vi "运维调试_质控单元.vi"() -> ()   [LabVIEW 2016, in "质控单元.lvlib"]
uses:
  <vilib>/Utility/miscctls.llb/LVPointTypeDef.ctl
  <vilib>/Utility/config.llb/Read Key (I32).vi
  <vilib>/Utility/config.llb/Read Key (Boolean).vi
  <vilib>/Utility/config.llb/Read Key (U32).vi
  <vilib>/Utility/config.llb/Write Key (I32).vi
  <vilib>/Utility/config.llb/Write Key (Boolean).vi
  <vilib>/Utility/config.llb/NI_LVConfig.lvlib
panel:
  in  "定时启动":bool
  out "CODCr母液浓度":dbl caption="加标母液浓度" format="%.2f"
  out "CODCr加标水杯定容体积":dbl caption="加标水杯定容体积" format="%.2f"
  out "CODCr检出限":dbl caption="检出限" format="%.2f"
  out "CODCr量程":dbl caption="量程" format="%.2f"
  out "COD母液浓度":dbl caption="加标母液浓度" format="%.2f"
  out "COD加标水杯定容体积":dbl caption="加标水杯定容体积" format="%.2f"
  out "COD检出限":dbl caption="检出限" format="%.2f"
  out "COD量程":dbl caption="量程" format="%.2f"
  out "总氮母液浓度":dbl caption="加标母液浓度" format="%.3f"
  out "总氮加标水杯定容体积":dbl caption="加标水杯定容体积" format="%.2f"
  out "总氮检出限":dbl caption="检出限" format="%.3f"
  out "总氮量程":dbl caption="量程" format="%.2f"
  out "总磷母液浓度":dbl caption="加标母液浓度" format="%.3f"
  out "总磷加标水杯定容体积":dbl caption="加标水杯定容体积" format="%.2f"
  out "总磷检出限":dbl caption="检出限" format="%.3f"
  out "总磷量程":dbl caption="量程" format="%.2f"
  out "氨氮母液浓度":dbl caption="加标母液浓度" format="%.3f"
  out "氨氮加标水杯定容体积":dbl caption="加标水杯定容体积" format="%.2f"
  out "氨氮检出限":dbl caption="检出限" format="%.3f"
  out "氨氮量程":dbl caption="量程" format="%.2f"
  in  "释放串口":bool
  in  "打开串口":bool
  out "CODCr质控流程中":bool
  out "CODMn质控流程中":bool
  out "总磷质控流程中":bool
  out "总氮质控流程中":bool
  out "氨氮质控流程中":bool
  out "CODCr通讯":bool
  out "CODMn通讯":bool
  out "总磷总氮通讯":bool
  out "氨氮通讯":bool
  out "CODCr传感器状态显示":bool
  out "CODCr超时报警":bool
  out "CODMn超时报警":bool
  out "总磷总氮超时报警":bool
  out "氨氮进样超时报警":bool
  out "CODMn传感器状态显示":bool
  out "总磷总氮传感器状态显示":bool
  out "氨氮传感器状态显示":bool
  out "CODCr流程中断报警":bool
  out "总磷总氮流程中断报警":bool
  out "CODMn流程中断报警":bool
  out "氨氮流程中断报警":bool
  in  "手动调试":bool
  in  "报警清除":bool
  in  "查看":bool
  in  "停止测量":bool
  in  "加标回收":bool
  in  "平行样测试":bool
  in  "CODCr量程选择":enum32{"H", "L", "AUTO"}(ring)
  in  "CODCr选择":bool
  out "CODCr加标回收率":dbl caption="加标回收率" format="%.2f"
  out "CODCr加标体积":dbl caption="加标体积" format="%.3f"
  out "CODCr加标后水样浓度":dbl caption="加标后水样浓度" format="%.2f"
  out "CODCr加标前水样浓度":dbl caption="加标前水样浓度" format="%.2f"
  out "CODCr状态":u16(ring) caption="状态" items=["待机", "润洗", "进样", "等待取液", "排液"]
  out "质控流程中":bool
  in  "CODMn量程选择":enum32{"H", "L", "AUTO"}(ring)
  in  "总磷量程选择":enum32{"H", "L", "AUTO"}(ring)=enum."AUTO"
  in  "总氮量程选择":enum32{"H", "L", "AUTO"}(ring)=enum."AUTO"
  in  "氨氮量程选择":enum32{"H", "L", "AUTO"}(ring)=enum."AUTO"
  in  "CODMn选择":bool
  in  "总磷总氮模块选择":bool
  in  "氨氮模块":bool
  in  "背隙补偿步数 3":i32 min=0 max=2000
  in  "背隙补偿步数 2":i32 min=0 max=2000
  in  "背隙补偿步数":i32 min=0 max=2000
  out "总氮加标回收率":dbl caption="加标回收率" format="%.2f"
  out "总氮加标体积":dbl caption="加标体积" format="%.3f"
  out "总氮加标后水样浓度":dbl caption="加标后水样浓度" format="%.3f"
  out "总氮加标前水样浓度":dbl caption="加标前水样浓度" format="%.3f"
  out "总氮状态":u16(ring) caption="状态" items=["待机", "润洗", "进样", "等待取液", "排液"]
  in  "返回":bool
  out "COD加标回收率":dbl caption="加标回收率" format="%.2f"
  out "COD加标体积":dbl caption="加标体积" format="%.3f"
  out "COD加标后水样浓度":dbl caption="加标后水样浓度" format="%.2f"
  out "COD加标前水样浓度":dbl caption="加标前水样浓度" format="%.2f"
  out "CODMn状态":u16(ring) caption="状态" items=["待机", "润洗", "进样", "等待取液", "排液"]
  out "总磷加标回收率":dbl caption="加标回收率" format="%.2f"
  out "总磷加标体积":dbl caption="加标体积" format="%.3f"
  out "总磷加标后水样浓度":dbl caption="加标后水样浓度" format="%.3f"
  out "总磷加标前水样浓度":dbl caption="加标前水样浓度" format="%.3f"
  out "总磷状态":u16(ring) caption="状态" items=["待机", "润洗", "进样", "等待取液", "排液"]
  out "氨氮加标回收率":dbl caption="加标回收率" format="%.2f"
  out "氨氮加标体积":dbl caption="加标体积" format="%.3f"
  out "氨氮加标后水样浓度":dbl caption="加标后水样浓度" format="%.3f"
  out "氨氮加标前水样浓度":dbl caption="加标前水样浓度" format="%.3f"
  out "氨氮状态":u16(ring) caption="状态" items=["待机", "润洗", "进样", "等待取液", "排液"]
  # "氨氮"
  # "总磷"
  # "总氮"
  # "CODMn"
  # "CODCr"
  # "参数配置区"
  # "2000步等于1mL\n100步等于0.05mL\n20步等于0.01mL\n2步等于0.001mL\n（初始默认100步）"
  # "CODCr质控参数"
  # "mg/L"
  # "mL"
  # "mg/L"
  # "mg/L"
  # "CODMn质控参数"
  # "mg/L"
  # "mL"
  # "mg/L"
  # "mg/L"
  # "总氮质控参数"
  # "mg/L"
  # "mL"
  # "mg/L"
  # "mg/L"
  # "总磷质控参数"
  # "mg/L"
  # "mL"
  # "mg/L"
  # "mg/L"
  # "氨氮质控参数"
  # "mg/L"
  # "mL"
  # "mg/L"
  # "mg/L"
  # "%"
  # "mL"
  # "mg/L"
  # "mg/L"
  # "%"
  # "mL"
  # "mg/L"
  # "mg/L"
  # "%"
  # "mL"
  # "mg/L"
  # "mg/L"
  # "%"
  # "mL"
  # "mg/L"
  # "mg/L"
  # "%"
  # "mL"
  # "mg/L"
  # "mg/L"
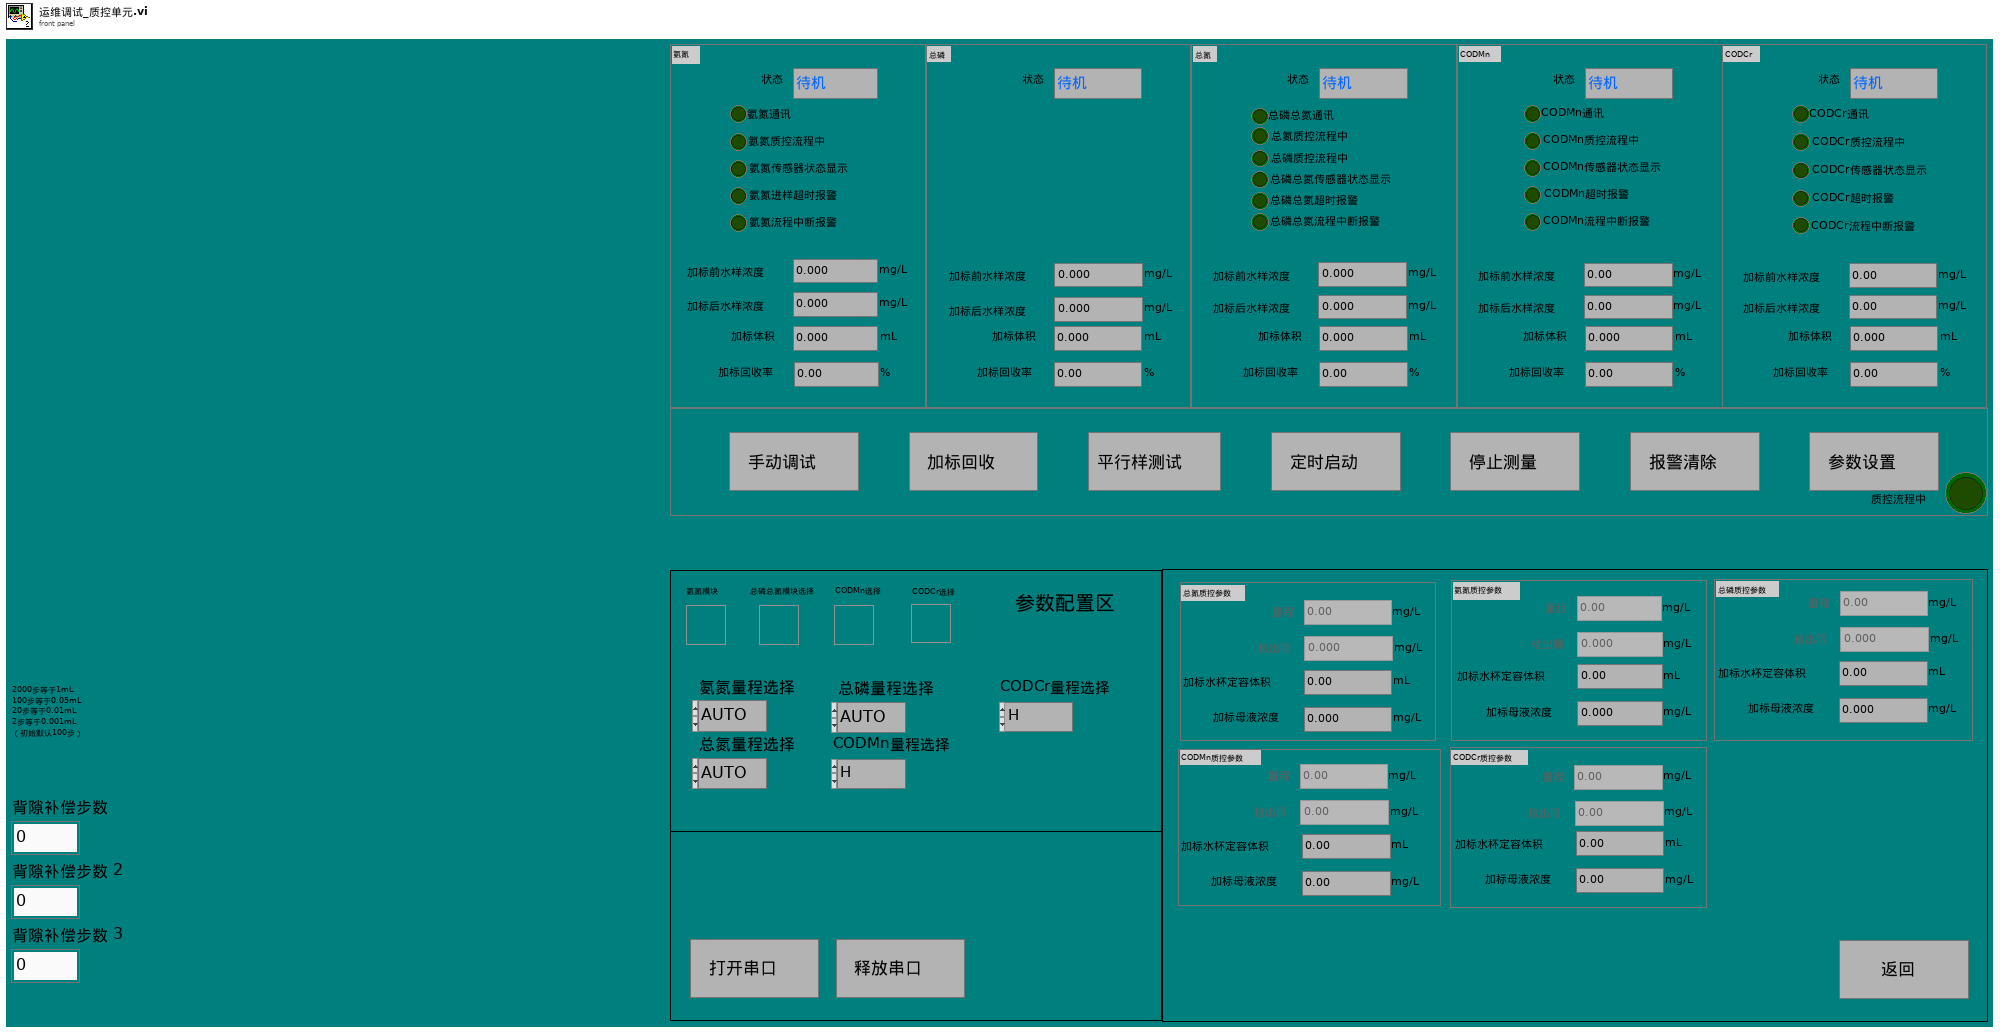
[diagram p1: front panel]
types:
  T1 = typedef "LVPointTypeDef.ctl" = cluster{"Horizontal":i16, "Vertical":i16}
  T2 = typedef "NI_LVConfig.lvlib/Config Data RefNum.ctl" = refnum<k1>
  T3 = cluster{"量程":dbl, "检出限":dbl, "加标前水样浓度":dbl, "加标后水样浓度":dbl, "加标水杯定容体积":dbl, "加标母液浓度":dbl, "加标体积":dbl, "加标回收率":dbl}
  T4 = enum8{"Enabled", "Disabled", "Disabled and Grayed Out"}
  T5 = cluster{"是否启用仪器":bool, "CODMn":cluster{"启动测量模式":cluster{"测量模式":enum16{"水样测量", "标样核查", "加标回收", "平行样", "校零", "校标"}}, "确定按钮":bool}, "启动模块":cluster{"氨氮":bool, "总磷":bool, "总氮":bool, "CODMn":bool, "CODCr":bool}, "常规启动":bool, "直接启动":bool}
  T6 = cluster{"参数启用":cluster{"CODMn":bool, "总磷":bool, "总氮":bool, "氨氮":bool, "CODcr":bool}, "采配水是否启动":bool}
  T7 = cluster{"命令":string, cluster{"starting address":u16, "holding register value":u16}}
  T8 = cluster{"周期设置类型":enum16{"定点启动", "间隔启动"}, "定时功能启用":bool, "定时间隔":dbl, "间隔启动次数 ":dbl, "已经启动次数 ":dbl, "24H周期设置":bool[], "模块选择":cluster{"氨氮":bool, "总磷":bool, "总氮":bool, "CODMn":bool, "CODCr":bool}, "采配水启用":bool}
  T9 = cluster{"周期设置类型":enum16{"定点启动", "间隔启动"}, "定时功能启用":bool, "定时间隔":dbl, "间隔启动次数":dbl, "已经启动次数":dbl, "24H周期设置":bool[], "模块选择":cluster{"氨氮":bool, "总磷":bool, "总氮":bool, "CODMn":bool, "CODCr":bool}, "采配水启用":bool}
  T10 = cluster{"氨氮":bool, "总磷":bool, "总氮":bool, "CODMn":bool, "CODCr":bool}
  T11 = enum32{"Bad", "Idle", "Run top level", "Running"}
  T12 = cluster{"CODMn":bool, "总磷":bool, "总氮":bool, "氨氮":bool, "CODCr":bool}
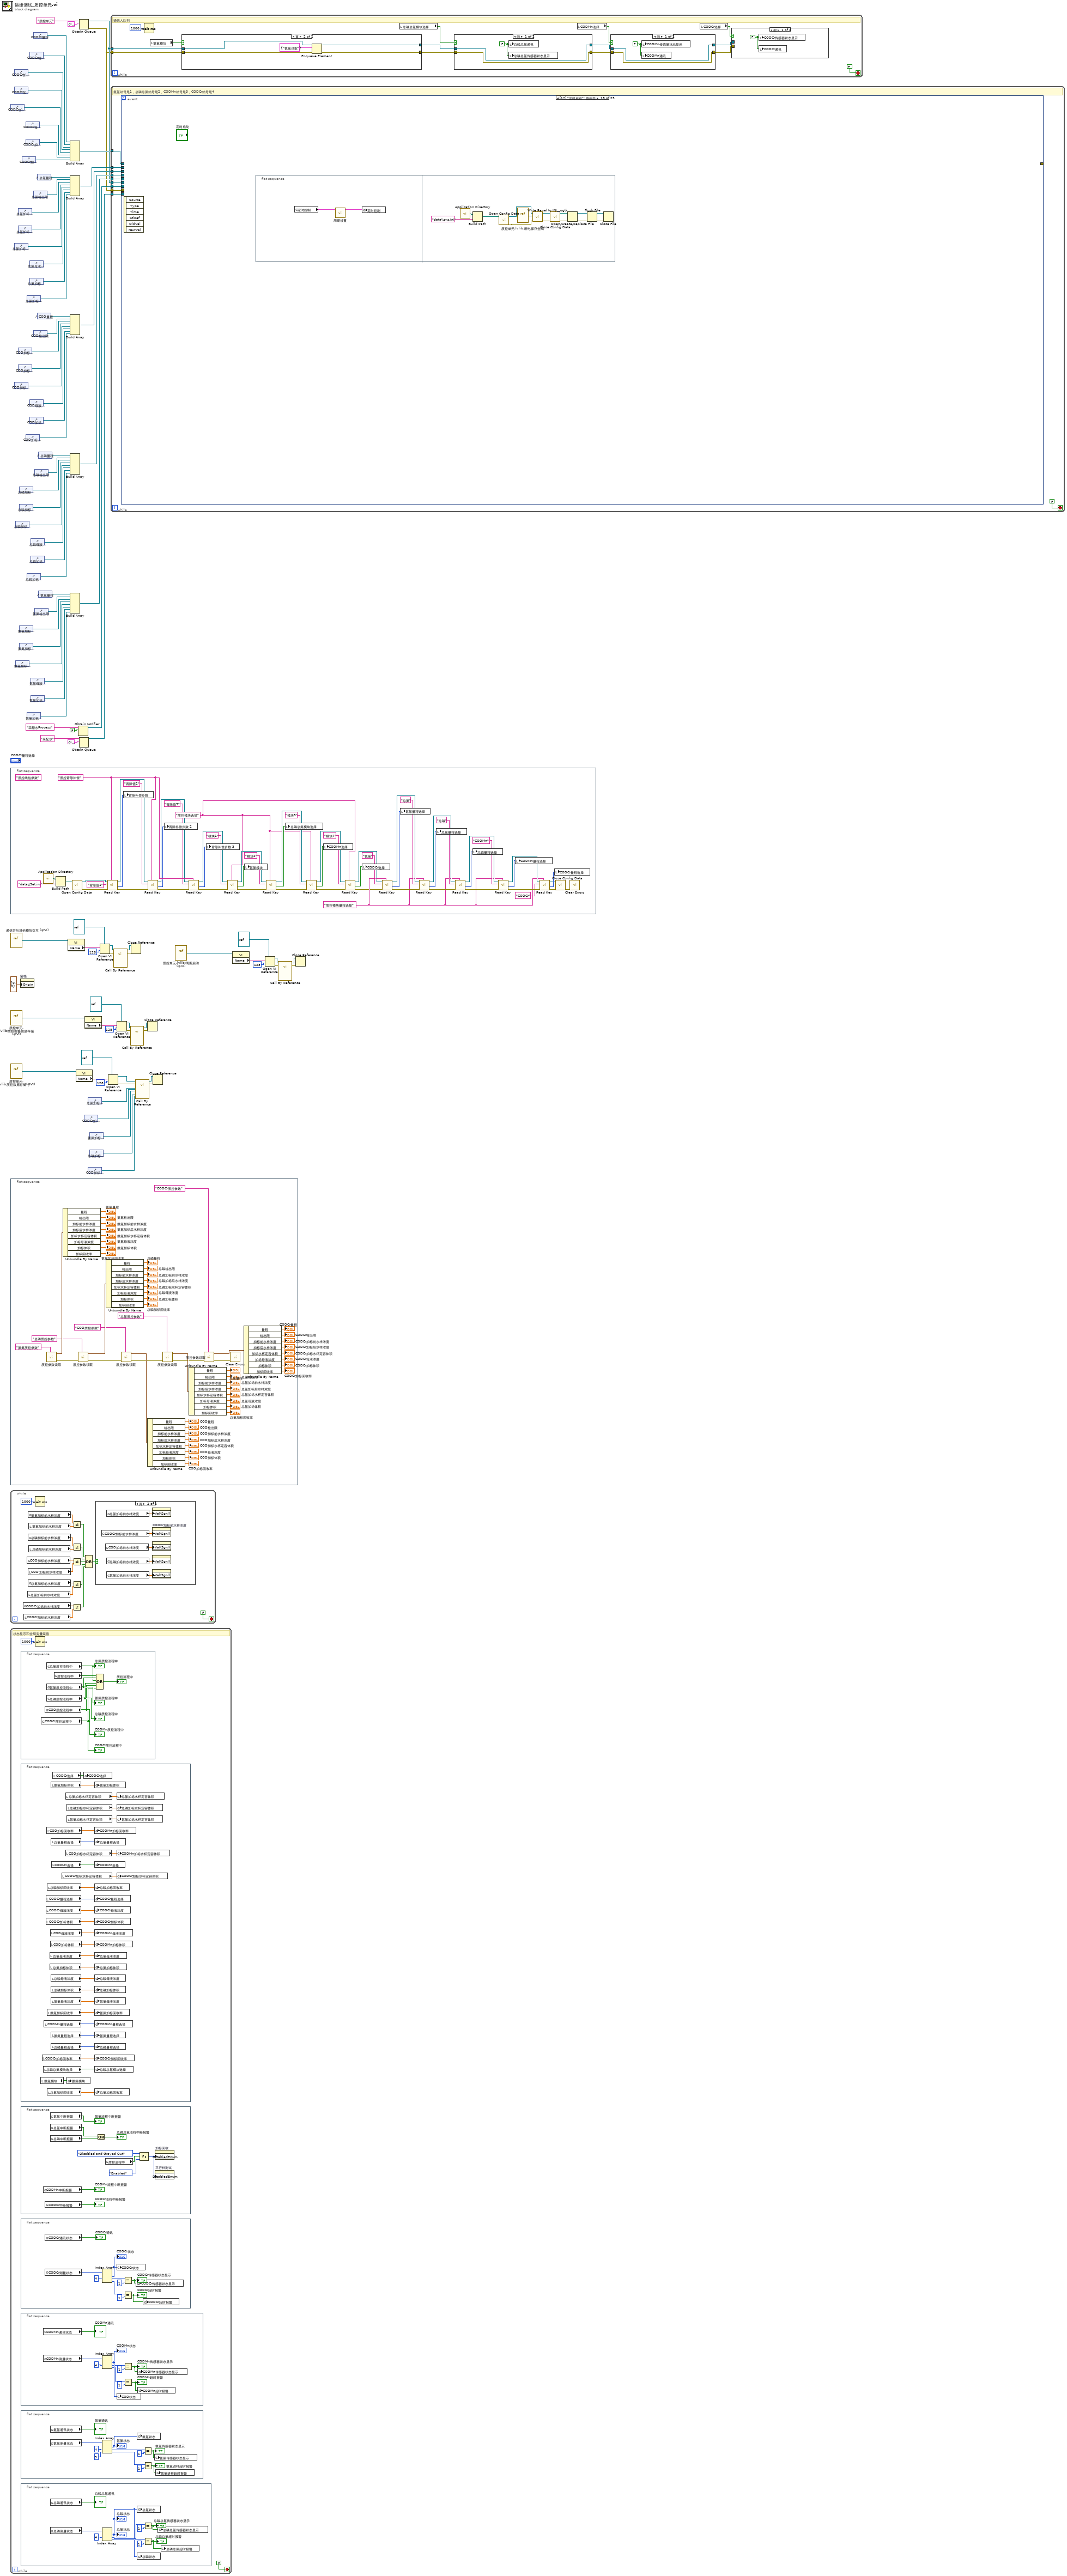
[diagram p0: block diagram]
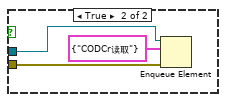
[diagram p2: hidden frame]
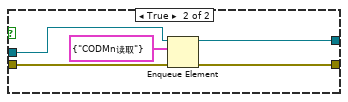
[diagram p3: hidden frame]
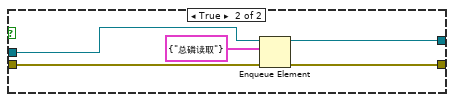
[diagram p4: hidden frame]
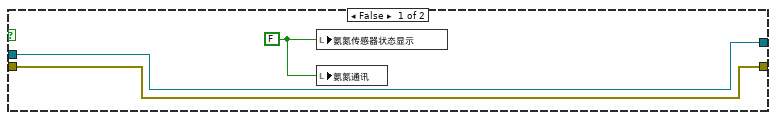
[diagram p5: hidden frame]
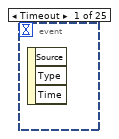
[diagram p7: hidden frame]
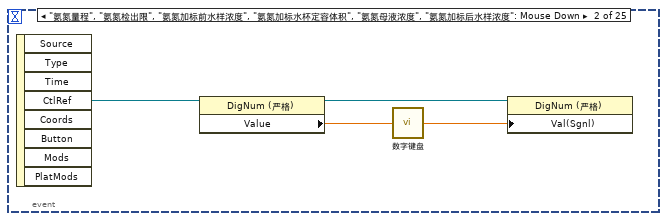
[diagram p8: hidden frame]
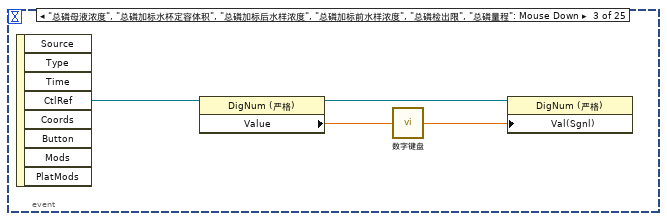
[diagram p9: hidden frame]
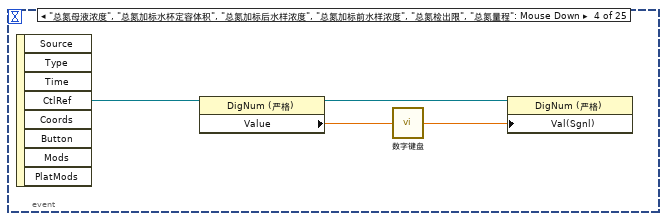
[diagram p10: hidden frame]
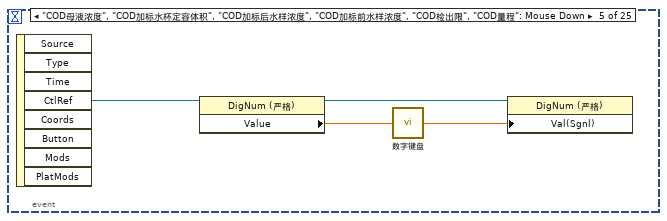
[diagram p11: hidden frame]
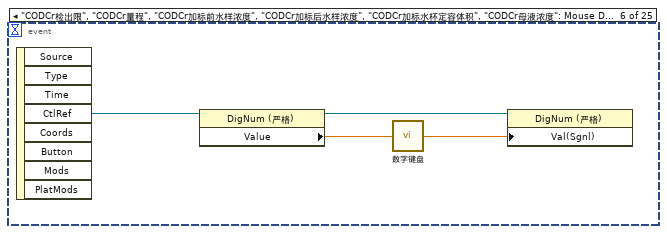
[diagram p12: hidden frame]
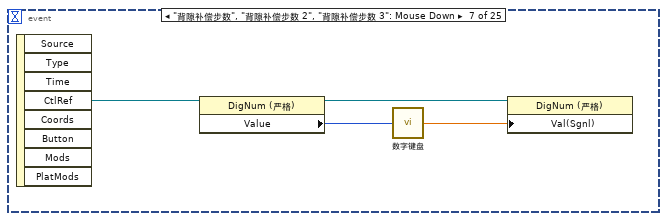
[diagram p13: hidden frame]
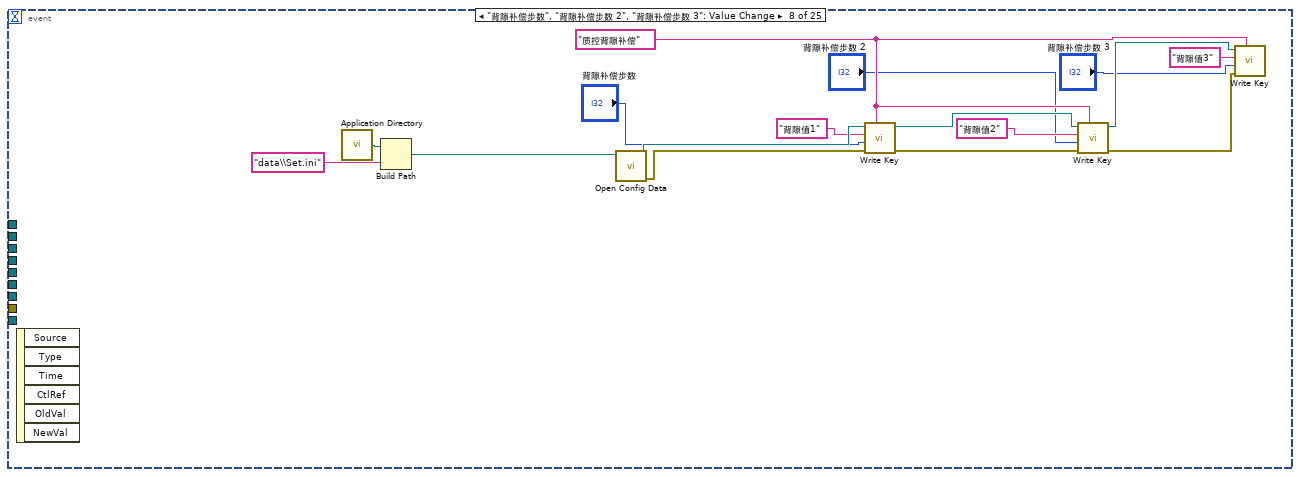
[diagram p14: hidden frame]
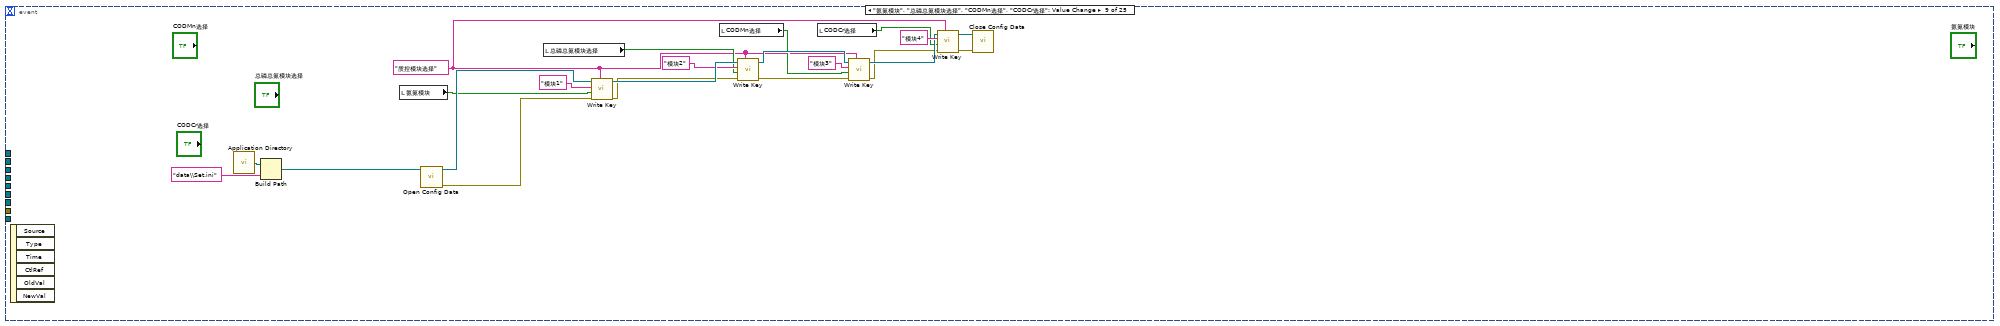
[diagram p15: hidden frame]
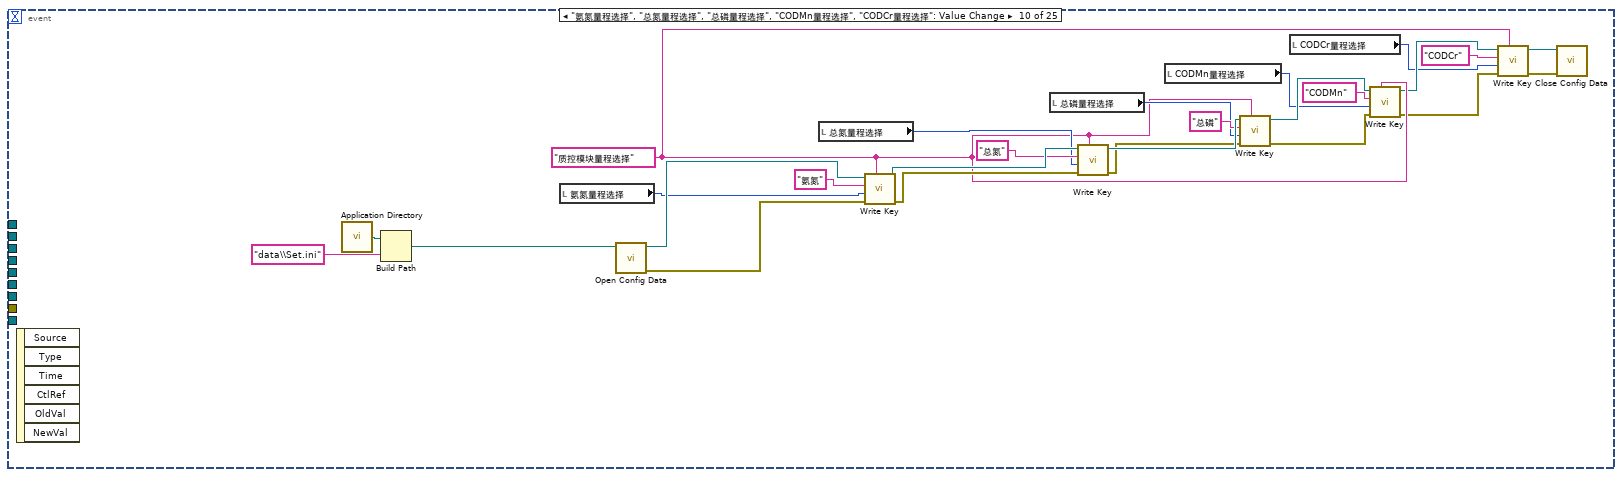
[diagram p16: hidden frame]
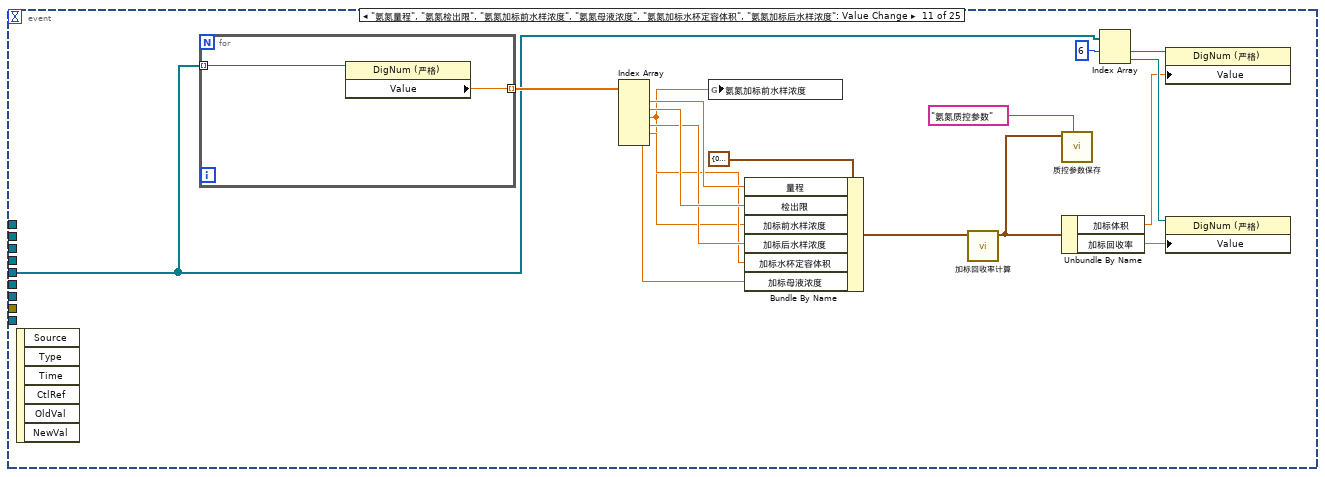
[diagram p17: hidden frame]
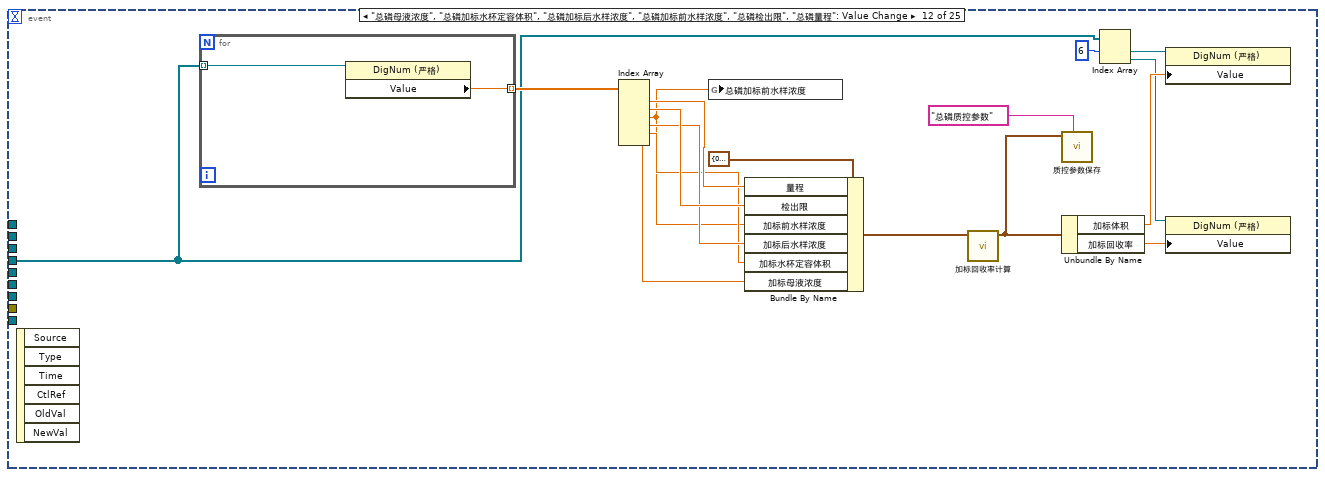
[diagram p18: hidden frame]
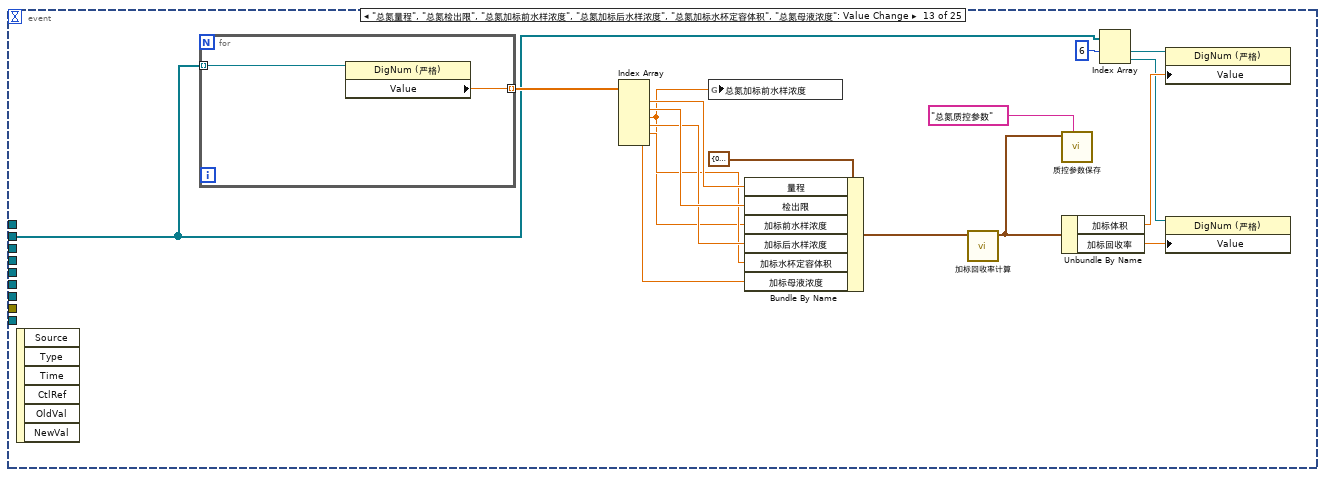
[diagram p19: hidden frame]
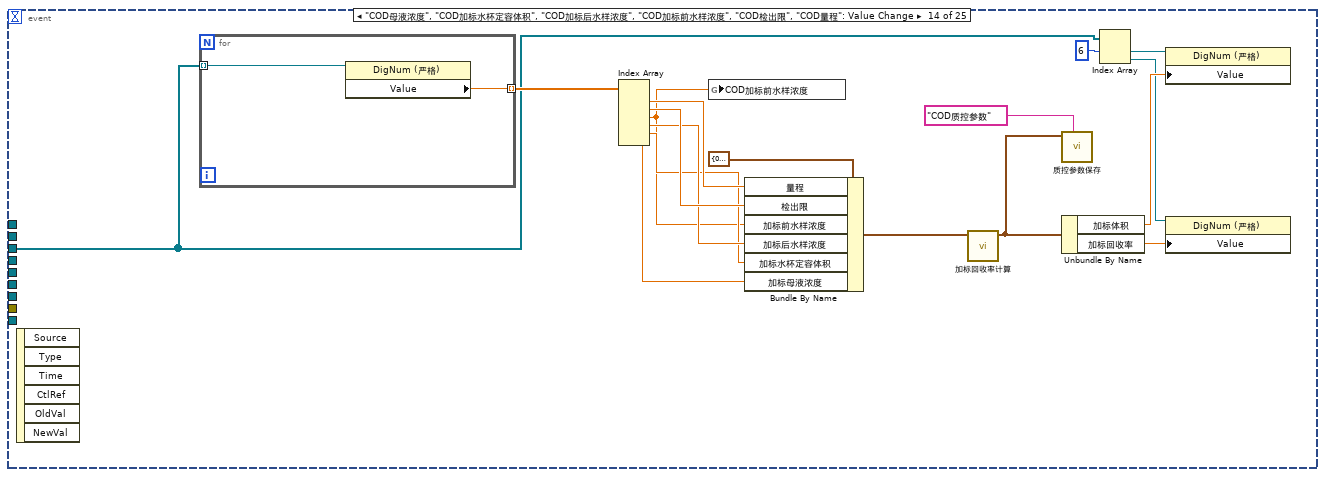
[diagram p20: hidden frame]
diagram:
  n1 = control-ref of="CODCr加标水杯定容体积"() -> (w46:refnum<vi>)
  n2 = flat-sequence {
    frame #0 {
      w108 = "质控模块量程选择" ("section")
      w100 = "质控模块选择" ("section")
      (unwired) "质控线性参数" ("section")
      w144 = "质控背隙补偿" ("section")
      n3 = call <vilib>:"Application Directory.vi"() -> ("Application Directory"=w150:path)
      n4 = Build Path(base path=w150, name or relative path="data\\Set.ini" ("名称或相对路径")) -> (appended path=w148:path)
      n5 = call <vilib>:"Open Config Data.vi"("configuration file path"=w148) -> ("error out"=w146:errorcluster, "refnum"=w147:T2)  [unwired: 8 in, 1 out]
      n6 = call-poly <vilib>:"Read Key.vi"("section"=w144, "error in (no error)"=w146, "key"="背隙值1", "refnum"=w147) -> ("error out"=w141:errorcluster, "value"=w136:i32, "refnum out"=w143:T2)  [unwired: 4 in, 1 out]
      n7 = local write "背隙补偿步数"(w136) -> ()
      n8 = call-poly <vilib>:"Read Key.vi"("section"=w144, "error in (no error)"=w141, "key"="背隙值2", "refnum"=w143) -> ("error out"=w139:errorcluster, "value"=w137:i32, "refnum out"=w140:T2)  [unwired: 4 in, 1 out]
      n9 = local write "背隙补偿步数 2"(w137) -> ()
      n10 = call-poly <vilib>:"Read Key.vi"("section"=w144, "error in (no error)"=w139, "key"="背隙值3", "refnum"=w140) -> ("error out"=w95:errorcluster, "value"=w135:i32, "refnum out"=w96:T2)  [unwired: 4 in, 1 out]
      n11 = local write "背隙补偿步数 3"(w135) -> ()
      n12 = call-poly <vilib>:"Read Key.vi"("section"=w100, "error in (no error)"=w95, "key"="模块1" ("section"), "refnum"=w96) -> ("error out"=w133:errorcluster, "value"=w125:bool, "refnum out"=w134:T2)  [unwired: 4 in, 1 out]
      n13 = local write "氨氮模块"(w125) -> ()
      n14 = call-poly <vilib>:"Read Key.vi"("section"=w100, "error in (no error)"=w133, "key"="模块2" ("section"), "refnum"=w134) -> ("error out"=w131:errorcluster, "value"=w126:bool, "refnum out"=w132:T2)  [unwired: 4 in, 1 out]
      n15 = local write "总磷总氮模块选择"(w126) -> ()
      n16 = call-poly <vilib>:"Read Key.vi"("section"=w100, "error in (no error)"=w131, "key"="模块3" ("section"), "refnum"=w132) -> ("error out"=w102:errorcluster, "value"=w127:bool, "refnum out"=w103:T2)  [unwired: 4 in, 1 out]
      n17 = local write "CODMn选择"(w127) -> ()
      n18 = call-poly <vilib>:"Read Key.vi"("section"=w100, "error in (no error)"=w102, "key"="模块4", "refnum"=w103) -> ("error out"=w98:errorcluster, "value"=w97:bool, "refnum out"=w99:T2)  [unwired: 4 in, 1 out]
      n19 = local write "CODCr选择"(w97) -> ()
      n20 = call-poly <vilib>:"Read Key.vi"("section"=w108, "error in (no error)"=w98, "key"="氨氮" ("section"), "refnum"=w99) -> ("error out"=w123:errorcluster, "value"=w114:u32, "refnum out"=w124:T2)  [unwired: 4 in, 1 out]
      n21 = local write "氨氮量程选择"(w114) -> ()
      n22 = call-poly <vilib>:"Read Key.vi"("section"=w108, "error in (no error)"=w123, "key"="总氮" ("section"), "refnum"=w124) -> ("error out"=w121:errorcluster, "value"=w113:u32, "refnum out"=w122:T2)  [unwired: 4 in, 1 out]
      n23 = local write "总氮量程选择"(w113) -> ()
      n24 = call-poly <vilib>:"Read Key.vi"("section"=w108, "error in (no error)"=w121, "key"="总磷" ("section"), "refnum"=w122) -> ("error out"=w119:errorcluster, "value"=w112:u32, "refnum out"=w120:T2)  [unwired: 4 in, 1 out]
      n25 = local write "总磷量程选择"(w112) -> ()
      n26 = call-poly <vilib>:"Read Key.vi"("section"=w108, "error in (no error)"=w119, "key"="CODMn" ("section"), "refnum"=w120) -> ("error out"=w109:errorcluster, "value"=w111:u32, "refnum out"=w110:T2)  [unwired: 4 in, 1 out]
      n27 = local write "CODMn量程选择"(w111) -> ()
      n28 = call-poly <vilib>:"Read Key.vi"("section"=w108, "error in (no error)"=w109, "key"="CODCr" ("section"), "refnum"=w110) -> ("error out"=w105:errorcluster, "value"=w106:u32, "refnum out"=w104:T2)  [unwired: 4 in, 1 out]
      n29 = local write "CODCr量程选择"(w106) -> ()
      n30 = call <vilib>:"Close Config Data.vi"("error in (no error)"=w105, "refnum"=w104) -> ("error out"=w94:errorcluster)  [unwired: 8 in, 1 out]
      n31 = call <vilib>:"Clear Errors.vi"("error in (no error)"=w94) -> ()  [unwired: 5 in, 2 out]
    }
  }
  n32 = vi-ref "通信并与其他模块交互 (子VI).vi"() -> (w34:refnum<vi>)
  n33 = vi-ref "质控单元.lvlib:质控报警信息存储 (子VI).vi"() -> (w29:refnum<vi>)
  n34 = vi-ref "质控单元.lvlib:质控数据存储(子VI).vi"() -> (w14:refnum<vi>)
  n35 = flat-sequence {
    frame #0 {
      n36 = call "质控参数读取.vi"("section"="氨氮质控参数") -> ("error out"=w185:errorcluster, "参数"=w204:T3)  [unwired: 9 in]
      n37 = Unbundle By Name(w204) -> ("量程"=→"氨氮量程":dbl, "检出限"=→"氨氮检出限":dbl, "加标前水样浓度"=→"氨氮加标前水样浓度":dbl, "加标后水样浓度"=→"氨氮加标后水样浓度":dbl, "加标水杯定容体积"=→"氨氮加标水杯定容体积":dbl, "加标母液浓度"=→"氨氮母液浓度":dbl, "加标体积"=→"氨氮加标体积":dbl, "加标回收率"=→"氨氮加标回收率":dbl)
      n38 = call "质控参数读取.vi"("section"="总磷质控参数", "error in (no error)"=w185) -> ("error out"=w182:errorcluster, "参数"=w194:T3)  [unwired: 8 in]
      n39 = Unbundle By Name(w194) -> ("量程"=→"总磷量程":dbl, "检出限"=→"总磷检出限":dbl, "加标前水样浓度"=→"总磷加标前水样浓度":dbl, "加标后水样浓度"=→"总磷加标后水样浓度":dbl, "加标水杯定容体积"=→"总磷加标水杯定容体积":dbl, "加标母液浓度"=→"总磷母液浓度":dbl, "加标体积"=→"总磷加标体积":dbl, "加标回收率"=→"总磷加标回收率":dbl)
      n40 = call "质控参数读取.vi"("section"="COD质控参数", "error in (no error)"=w182) -> ("error out"=w172:errorcluster, "参数"=w184:T3)  [unwired: 8 in]
      n41 = Unbundle By Name(w184) -> ("量程"=→"COD量程":dbl, "检出限"=→"COD检出限":dbl, "加标前水样浓度"=→"COD加标前水样浓度":dbl, "加标后水样浓度"=→"COD加标后水样浓度":dbl, "加标水杯定容体积"=→"COD加标水杯定容体积":dbl, "加标母液浓度"=→"COD母液浓度":dbl, "加标体积"=→"COD加标体积":dbl, "加标回收率"=→"COD加标回收率":dbl)
      n42 = call "质控参数读取.vi"("section"="总氮质控参数", "error in (no error)"=w172) -> ("error out"=w160:errorcluster, "参数"=w171:T3)  [unwired: 8 in]
      n43 = Unbundle By Name(w171) -> ("量程"=→"总氮量程":dbl, "检出限"=→"总氮检出限":dbl, "加标前水样浓度"=→"总氮加标前水样浓度":dbl, "加标后水样浓度"=→"总氮加标后水样浓度":dbl, "加标水杯定容体积"=→"总氮加标水杯定容体积":dbl, "加标母液浓度"=→"总氮母液浓度":dbl, "加标体积"=→"总氮加标体积":dbl, "加标回收率"=→"总氮加标回收率":dbl)
      n44 = call "质控参数读取.vi"("section"="CODCr质控参数", "error in (no error)"=w160) -> ("error out"=w151:errorcluster, "参数"=w161:T3)  [unwired: 8 in]
      n45 = call <vilib>:"Clear Errors.vi"("error in (no error)"=w151) -> ()  [unwired: 5 in, 2 out]
      n46 = Unbundle By Name(w161) -> ("量程"=→"CODCr量程":dbl, "检出限"=→"CODCr检出限":dbl, "加标前水样浓度"=→"CODCr加标前水样浓度":dbl, "加标后水样浓度"=→"CODCr加标后水样浓度":dbl, "加标水杯定容体积"=→"CODCr加标水杯定容体积":dbl, "加标母液浓度"=→"CODCr母液浓度":dbl, "加标体积"=→"CODCr加标体积":dbl, "加标回收率"=→"CODCr加标回收率":dbl)
    }
  }
  n47 = while {
    stop <- FALSE stop-if-true
    n48 = global read "水样浓度全局.vi" "CODCr加标前水样浓度"() -> (w208:dbl)
    n49 = local read "CODCr加标前水样浓度"() -> (w207:dbl)
    n50 = global read "水样浓度全局.vi" "COD加标前水样浓度"() -> (w217:dbl)
    n51 = local read "总氮加标前水样浓度"() -> (w211:dbl)
    n52 = global read "水样浓度全局.vi" "氨氮加标前水样浓度"() -> (w221:dbl)
    n53 = global read "水样浓度全局.vi" "总磷加标前水样浓度"() -> (w219:dbl)
    n54 = local read "COD加标前水样浓度"() -> (w216:dbl)
    n55 = global read "水样浓度全局.vi" "总氮加标前水样浓度"() -> (w210:dbl)
    n56 = local read "氨氮加标前水样浓度"() -> (w220:dbl)
    n57 = local read "总磷加标前水样浓度"() -> (w218:dbl)
    n58 = Wait (ms)(milliseconds to wait=u32 1000 ("等待时间（毫秒）")) -> ()  [unwired: 1 out]
    n59 = Not Equal?(x=w221, y=w220) -> (x != y?=w215:bool)
    n60 = Not Equal?(x=w219, y=w218) -> (x != y?=w213:bool)
    n61 = Not Equal?(x=w217, y=w216) -> (x != y?=w212:bool)
    n62 = Not Equal?(x=w210, y=w211) -> (x != y?=w209:bool)
    n63 = Not Equal?(x=w208, y=w207) -> (x != y?=w206:bool)
    n64 = Compound Arithmetic op=OR ("复合运算")(w215, w213, w212, w209, w206) -> (w214:bool)
    n65 = case shown="真" w214 {
      frame False {
      }
      frame True {
        n66 = global read "水样浓度全局.vi" "CODCr加标前水样浓度"() -> (w224:dbl)
        n67 = global read "水样浓度全局.vi" "COD加标前水样浓度"() -> (w226:dbl)
        n68 = global read "水样浓度全局.vi" "总氮加标前水样浓度"() -> (w225:dbl)
        n69 = global read "水样浓度全局.vi" "总磷加标前水样浓度"() -> (w227:dbl)
        n70 = global read "水样浓度全局.vi" "氨氮加标前水样浓度"() -> (w228:dbl)
        n71 = property on="总氮加标前水样浓度" class="DigNum (严格)"("Val(Sgnl)"=w225) -> ()  [unwired: 2 in, 2 out]
        n72 = property on="CODCr加标前水样浓度" class="DigNum (严格)"("Val(Sgnl)"=w224) -> ()  [unwired: 2 in, 2 out]
        n73 = property on="COD加标前水样浓度" class="DigNum (严格)"("Val(Sgnl)"=w226) -> ()  [unwired: 2 in, 2 out]
        n74 = property on="总磷加标前水样浓度" class="DigNum (严格)"("Val(Sgnl)"=w227) -> ()  [unwired: 2 in, 2 out]
        n75 = property on="氨氮加标前水样浓度" class="DigNum (严格)"("Val(Sgnl)"=w228) -> ()  [unwired: 2 in, 2 out]
      }
    }
  }
  n76 = while {
    stop <- FALSE stop-if-true
    # "状态显示和全局变量赋值"
    n77 = flat-sequence {
      frame #0 {
        n78 = global read "质控测完标志全局 1.vi" "CODCr质控流程中"() -> (w311:bool)
        "CODCr质控流程中" <- w311
        n79 = global read "质控测完标志全局 1.vi" "COD质控流程中"() -> (w312:bool)
        "CODMn质控流程中" <- w312
        n80 = global read "质控测完标志全局 1.vi" "总氮质控流程中"() -> (w314:bool)
        "总氮质控流程中" <- w314
        n81 = global read "质控测完标志全局 1.vi" "氨氮质控流程中"() -> (w315:bool)
        "氨氮质控流程中" <- w315
        n82 = global read "质控测完标志全局 1.vi" "总磷质控流程中"() -> (w313:bool)
        "总磷质控流程中" <- w313
        n83 = global read "质控测完标志全局 1.vi" "质控流程中"() -> (w317:bool)
        n84 = Compound Arithmetic op=OR ("复合运算")(w317, w315, w314, w313, w312, w311) -> (→"质控流程中":bool)
      }
    }
    n85 = flat-sequence {
      frame #0 {
        n86 = local read "氨氮模块"() -> (w305:bool)
        n87 = local read "CODCr加标回收率"() -> (w286:dbl)
        n88 = local read "总磷总氮模块选择"() -> (w304:bool)
        n89 = local read "CODMn量程选择"() -> (w309:enum32{"H", "L", "AUTO"})
        n90 = local read "CODCr量程选择"() -> (w310:enum32{"H", "L", "AUTO"})
        n91 = local read "CODCr母液浓度"() -> (w287:dbl)
        n92 = local read "CODCr加标体积"() -> (w297:dbl)
        n93 = local read "COD加标回收率"() -> (w285:dbl)
        n94 = local read "总磷加标回收率"() -> (w283:dbl)
        n95 = local read "氨氮加标回收率"() -> (w282:dbl)
        n96 = local read "总氮加标回收率"() -> (w284:dbl)
        n97 = local read "总氮母液浓度"() -> (w289:dbl)
        n98 = local read "总氮加标体积"() -> (w299:dbl)
        n99 = local read "COD母液浓度"() -> (w288:dbl)
        n100 = local read "COD加标体积"() -> (w298:dbl)
        n101 = local read "氨氮加标体积"() -> (w301:dbl)
        n102 = local read "总氮量程选择"() -> (w307:enum32{"H", "L", "AUTO"})
        n103 = local read "总磷母液浓度"() -> (w290:dbl)
        n104 = local read "总磷加标体积"() -> (w300:dbl)
        n105 = local read "氨氮母液浓度"() -> (w291:dbl)
        n106 = local read "氨氮量程选择"() -> (w308:enum32{"H", "L", "AUTO"})
        n107 = local read "总磷量程选择"() -> (w306:enum32{"H", "L", "AUTO"})
        n108 = local read "CODMn选择"() -> (w303:bool)
        n109 = local read "CODCr选择"() -> (w302:bool)
        n110 = local read "CODCr加标水杯定容体积"() -> (w296:dbl)
        n111 = local read "总氮加标水杯定容体积"() -> (w294:dbl)
        n112 = local read "COD加标水杯定容体积"() -> (w295:dbl)
        n113 = local read "总磷加标水杯定容体积"() -> (w293:dbl)
        n114 = local read "氨氮加标水杯定容体积"() -> (w292:dbl)
        n115 = global write "断电保存全局.vi" "氨氮模块"(w305) -> ()
        n116 = global write "断电保存全局.vi" "CODCr选择"(w302) -> ()
        n117 = global write "加标回收状态全局变量.vi" "氨氮加标体积"(w301) -> ()
        n118 = global write "加标回收状态全局变量.vi" "CODMn加标回收率"(w285) -> ()
        n119 = global write "断电保存全局.vi" "总氮量程选择"(w307) -> ()
        n120 = global write "断电保存全局.vi" "CODMn选择"(w303) -> ()
        n121 = global write "加标回收状态全局变量.vi" "总磷加标回收率"(w283) -> ()
        n122 = global write "断电保存全局.vi" "CODCr量程选择"(w310) -> ()
        n123 = global write "加标回收状态全局变量.vi" "CODCr母液浓度"(w287) -> ()
        n124 = global write "加标回收状态全局变量.vi" "CODCr加标体积"(w297) -> ()
        n125 = global write "加标回收状态全局变量.vi" "CODMn母液浓度"(w288) -> ()
        n126 = global write "加标回收状态全局变量.vi" "CODMn加标体积"(w298) -> ()
        n127 = global write "加标回收状态全局变量.vi" "总氮母液浓度"(w289) -> ()
        n128 = global write "加标回收状态全局变量.vi" "总氮加标体积"(w299) -> ()
        n129 = global write "加标回收状态全局变量.vi" "总磷母液浓度"(w290) -> ()
        n130 = global write "加标回收状态全局变量.vi" "总磷加标体积"(w300) -> ()
        n131 = global write "加标回收状态全局变量.vi" "氨氮母液浓度"(w291) -> ()
        n132 = global write "加标回收状态全局变量.vi" "氨氮加标回收率"(w282) -> ()
        n133 = global write "断电保存全局.vi" "CODMn量程选择"(w309) -> ()
        n134 = global write "断电保存全局.vi" "氨氮量程选择"(w308) -> ()
        n135 = global write "断电保存全局.vi" "总磷量程选择"(w306) -> ()
        n136 = global write "加标回收状态全局变量.vi" "CODCr加标回收率"(w286) -> ()
        n137 = global write "断电保存全局.vi" "总磷总氮模块选择"(w304) -> ()
        n138 = global write "加标回收状态全局变量.vi" "总氮加标回收率"(w284) -> ()
        n139 = global write "加标回收状态全局变量.vi" "总氮加标水杯定容体积"(w294) -> ()
        n140 = global write "加标回收状态全局变量.vi" "总磷加标水杯定容体积"(w293) -> ()
        n141 = global write "加标回收状态全局变量.vi" "氨氮加标水杯定容体积"(w292) -> ()
        n142 = global write "加标回收状态全局变量.vi" "CODMn加标水杯定容体积"(w295) -> ()
        n143 = global write "加标回收状态全局变量.vi" "CODCr加标水杯定容体积"(w296) -> ()
      }
    }
    n144 = flat-sequence {
      frame #0 {
        n145 = global read "质控中断报警全局.vi" "CODMn中断报警"() -> (→"CODMn流程中断报警":bool)
        n146 = global read "质控中断报警全局.vi" "CODCr中断报警"() -> (→"CODCr流程中断报警":bool)
        n147 = global read "质控中断报警全局.vi" "氨氮中断报警"() -> (→"氨氮流程中断报警":bool)
        n148 = global read "质控中断报警全局.vi" "总氮中断报警"() -> (w272:bool)
        n149 = global read "质控中断报警全局.vi" "总磷中断报警"() -> (w280:bool)
        n150 = Or(x=w272, y=w280) -> (x .or. y?=→"总磷总氮流程中断报警":bool)
        n151 = global read "质控测完标志全局 1.vi" "质控流程中"() -> (w277:bool)
        n152 = Select(t=T4."Disabled and Grayed Out" ("禁用"), s=w277, f=T4."Enabled") -> (s? t:f=w276:T4)
        n153 = property on="加标回收" class="Bool"("DisabledEnum"=w276) -> ()  [unwired: 2 in, 2 out]
        n154 = property on="平行样测试" class="Bool"("DisabledEnum"=w276) -> ()  [unwired: 2 in, 2 out]
      }
    }
    n155 = flat-sequence {
      frame #0 {
        n156 = global read "质控内部交互全局.vi" "CODCr通讯状态"() -> (→"CODCr通讯":bool)
        n157 = global read "质控内部交互全局.vi" "CODCr测量状态"() -> (w238:u16[])
        n158 = Index Array(array=w238, index #2=4 ("索引")) -> (element #1=w239:u16, element #2=w234:u16, element #3=w233:u16)  [unwired: 2 in]
        "CODCr状态" <- w239
        n159 = global write "加标回收状态全局变量.vi" "CODCr状态"(w239) -> ()
        n160 = Equal?(x=w234, y=u16 1) -> (x = y?=w231:bool)
        "CODCr传感器状态显示" <- w231
        n161 = Equal?(x=w233, y=u16 1) -> (x = y?=w232:bool)
        "CODCr超时报警" <- w232
        n162 = global write "质控中断报警全局.vi" "CODCr传感器状态显示"(w231) -> ()
        n163 = global write "质控中断报警全局.vi" "CODCr超时报警"(w232) -> ()
      }
    }
    n164 = flat-sequence {
      frame #0 {
        n165 = global read "质控内部交互全局.vi" "CODMn通讯状态"() -> (→"CODMn通讯":bool)
        n166 = global read "质控内部交互全局.vi" "CODMn测量状态"() -> (w246:u16[])
        n167 = Index Array(array=w246, index #2=4 ("索引")) -> (element #1=w249:u16, element #2=w247:u16, element #3=w243:u16)  [unwired: 2 in]
        "CODMn状态" <- w249
        n168 = global write "加标回收状态全局变量.vi" "COD状态"(w249) -> ()
        n169 = Equal?(x=w247, y=u16 1) -> (x = y?=w242:bool)
        "CODMn传感器状态显示" <- w242
        n170 = Equal?(x=w243, y=u16 1) -> (x = y?=w241:bool)
        "CODMn超时报警" <- w241
        n171 = global write "质控中断报警全局.vi" "CODMn超时报警"(w241) -> ()
        n172 = global write "质控中断报警全局.vi" "CODMn传感器状态显示"(w242) -> ()
      }
    }
    n173 = flat-sequence {
      frame #0 {
        n174 = global read "质控内部交互全局.vi" "氨氮通讯状态"() -> (→"氨氮通讯":bool)
        n175 = global read "质控内部交互全局.vi" "氨氮测量状态"() -> (w266:u16[])
        n176 = Index Array(array=w266, index #2=4 ("索引"), index #3=5 ("索引")) -> (element #1=w267:u16, element #2=w270:u16, element #3=w263:u16)  [unwired: 1 in]
        "氨氮状态" <- w267
        n177 = global write "加标回收状态全局变量.vi" "氨氮状态"(w267) -> ()
        n178 = Equal?(x=w270, y=u16 1) -> (x = y?=w262:bool)
        "氨氮传感器状态显示" <- w262
        n179 = Equal?(x=w263, y=u16 1) -> (x = y?=w261:bool)
        "氨氮进样超时报警" <- w261
        n180 = global write "质控中断报警全局.vi" "氨氮传感器状态显示"(w262) -> ()
        n181 = global write "质控中断报警全局.vi" "氨氮进样超时报警"(w261) -> ()
      }
    }
    n182 = flat-sequence {
      frame #0 {
        n183 = global read "质控内部交互全局.vi" "总磷通讯状态"() -> (→"总磷总氮通讯":bool)
        n184 = global read "质控内部交互全局.vi" "总磷测量状态"() -> (w256:u16[])
        n185 = Index Array(array=w256, index #2=4 ("索引")) -> (element #1=w257:u16, element #2=w258:u16, element #3=w253:u16)  [unwired: 2 in]
        "总氮状态" <- w257
        "总磷状态" <- w257
        n186 = global write "加标回收状态全局变量.vi" "总氮状态"(w257) -> ()
        n187 = global write "加标回收状态全局变量.vi" "总磷状态"(w257) -> ()
        n188 = Equal?(x=w258, y=u16 1) -> (x = y?=w252:bool)
        "总磷总氮传感器状态显示" <- w252
        n189 = Equal?(x=w253, y=u16 1) -> (x = y?=w251:bool)
        "总磷总氮超时报警" <- w251
        n190 = global write "质控中断报警全局.vi" "总磷总氮传感器状态显示"(w252) -> ()
        n191 = global write "质控中断报警全局.vi" "总磷总氮超时报警"(w251) -> ()
      }
    }
    n192 = Wait (ms)(milliseconds to wait=u32 1000 ("等待时间（毫秒）")) -> ()  [unwired: 1 out]
  }
  n193 = control-ref of="CODCr加标前水样浓度"() -> (w48:refnum<vi>)
  n194 = control-ref of="CODCr加标后水样浓度"() -> (w47:refnum<vi>)
  n195 = control-ref of="总氮加标水杯定容体积"() -> (w55:refnum<vi>)
  n196 = control-ref of="COD加标水杯定容体积"() -> (w71:refnum<vi>)
  n197 = control-ref of="总磷加标水杯定容体积"() -> (w80:refnum<vi>)
  n198 = control-ref of="氨氮加标水杯定容体积"() -> (w90:refnum<vi>)
  n199 = control-ref of="总氮加标前水样浓度"() -> (w57:refnum<vi>)
  n200 = control-ref of="总氮加标后水样浓度"() -> (w56:refnum<vi>)
  n201 = control-ref of="COD加标前水样浓度"() -> (w73:refnum<vi>)
  n202 = control-ref of="COD加标后水样浓度"() -> (w72:refnum<vi>)
  n203 = control-ref of="总磷加标前水样浓度"() -> (w82:refnum<vi>)
  n204 = control-ref of="总磷加标后水样浓度"() -> (w81:refnum<vi>)
  n205 = control-ref of="氨氮加标前水样浓度"() -> (w91:refnum<vi>)
  n206 = control-ref of="氨氮加标后水样浓度"() -> (w87:refnum<vi>)
  n207 = property on="窗格" class="Pane"("Origin"=T1 {"Horizontal"=0, "Vertical"=0} ("原点")) -> ()  [unwired: 2 in, 2 out]
  n208 = control-ref of="CODCr加标回收率"() -> (w43:refnum<vi>)
  n209 = control-ref of="CODCr母液浓度"() -> (w45:refnum<vi>)
  n210 = control-ref of="CODCr加标体积"() -> (w44:refnum<vi>)
  n211 = control-ref of="COD加标回收率"() -> (w68:refnum<vi>)
  n212 = control-ref of="总氮加标回收率"() -> (w52:refnum<vi>)
  n213 = control-ref of="总磷加标回收率"() -> (w78:refnum<vi>)
  n214 = control-ref of="氨氮加标回收率"() -> (w85:refnum<vi>)
  n215 = control-ref of="CODCr检出限"() -> (w49:refnum<vi>)
  n216 = control-ref of="总氮母液浓度"() -> (w54:refnum<vi>)
  n217 = control-ref of="总氮加标体积"() -> (w53:refnum<vi>)
  n218 = control-ref of="COD母液浓度"() -> (w70:refnum<vi>)
  n219 = control-ref of="COD加标体积"() -> (w69:refnum<vi>)
  n220 = control-ref of="总磷母液浓度"() -> (w79:refnum<vi>)
  n221 = control-ref of="总磷加标体积"() -> (w77:refnum<vi>)
  n222 = control-ref of="氨氮母液浓度"() -> (w89:refnum<vi>)
  n223 = control-ref of="氨氮加标体积"() -> (w86:refnum<vi>)
  n224 = control-ref of="CODCr量程"() -> (w50:refnum<vi>)
  n225 = control-ref of="总氮检出限"() -> (w58:refnum<vi>)
  n226 = control-ref of="COD检出限"() -> (w74:refnum<vi>)
  n227 = control-ref of="总磷检出限"() -> (w83:refnum<vi>)
  n228 = control-ref of="氨氮检出限"() -> (w92:refnum<vi>)
  n229 = control-ref of="总氮量程"() -> (w59:refnum<vi>)
  n230 = control-ref of="COD量程"() -> (w75:refnum<vi>)
  n231 = control-ref of="总磷量程"() -> (w84:refnum<vi>)
  n232 = control-ref of="氨氮量程"() -> (w93:refnum<vi>)
  n233 = property class="VI"(reference=w34) -> ("Name"=w35:string)  [unwired: 1 in, 2 out]
  n234 = Build Array(w50, w49, w48, w47, w46, w45, w44, w43) -> (w42:refnum<vi>[])
  n235 = Build Array(w59, w58, w57, w56, w55, w54, w53, w52) -> (w51:refnum<vi>[])
  n236 = Build Array(w75, w74, w73, w72, w71, w70, w69, w68) -> (w67:refnum<vi>[])
  n237 = Build Array(w84, w83, w82, w81, w80, w79, w77, w78) -> (w76:refnum<vi>[])
  n238 = Build Array(w93, w92, w91, w87, w90, w89, w86, w85) -> (w88:refnum<vi>[])
  n239 = property class="VI"(reference=w14) -> ("Name"=w15:string)  [unwired: 1 in, 2 out]
  n240 = Obtain Notifier(name (unnamed)="采配水Process" ("名称（未命名）"), notification data type=FALSE) -> (notifier out=w64:refnum<notifier>)  [unwired: 2 in, 2 out]
  n241 = Obtain Queue(name (unnamed)="质控单元" ("名称（未命名）"), element data type=cluster{"命令":string} {"命令"="启用模块"} ("元素")) -> (queue out=w31:refnum<queue>, error out=w30:errorcluster)  [unwired: 3 in, 1 out]
  n242 = Obtain Queue(name (unnamed)="采配水" ("名称（未命名）"), element data type=cluster{"命令":string, "数据":variant} {"命令"="", "数据"=variant}) -> (queue out=w61:refnum<queue>)  [unwired: 3 in, 2 out]
  n243 = control-ref of="CODCr加标后水样浓度"() -> (w13:refnum<vi>)
  n244 = property class="VI"(reference=w29) -> ("Name"=w28:string)  [unwired: 1 in, 2 out]
  n245 = control-ref of="总氮加标后水样浓度"() -> (w12:refnum<vi>)
  n246 = control-ref of="COD加标后水样浓度"() -> (w9:refnum<vi>)
  n247 = control-ref of="氨氮加标后水样浓度"() -> (w11:refnum<vi>)
  n248 = control-ref of="总磷加标后水样浓度"() -> (w10:refnum<vi>)
  n249 = Open VI Reference(type specifier VI Refnum (for type only)=refnum<vi> refnum, vi path=w35, options=128 ("选项")) -> (vi reference=w37:refnum<vi>, error out=w39:errorcluster)  [unwired: 3 in]
  n250 = Open VI Reference(type specifier VI Refnum (for type only)=refnum<vi> refnum, vi path=w15, options=128 ("选项")) -> (vi reference=w17:refnum<vi>, error out=w19:errorcluster)  [unwired: 3 in]
  n251 = while {
    tunnel: w31 -> [w321]
    tunnel: w30 -> [w320]
    stop <- FALSE stop-if-true
    # "通信入队列"
    n252 = Wait (ms)(milliseconds to wait=u32 1000 ("等待时间（毫秒）")) -> ()  [unwired: 1 out]
    n253 = local read "氨氮模块"() -> (w322:bool)
    n254 = case shown="真" w322 {
      tunnel: w321 -> [w353 w358]
      tunnel: w320 -> [w352 w357]
      tunnel: [w353 w356] -> w326
      tunnel: [w352 w355] -> w327
      frame False {
        w354 = FALSE ("通讯指示灯1")
        n255 = local write "氨氮传感器状态显示"(w354) -> ()
        n256 = local write "氨氮通讯"(w354) -> ()
      }
      frame True {
        n257 = Enqueue Element(queue=w358, element=cluster{"命令":string} {"命令"="氨氮读取"} ("元素"), error in (no error)=w357) -> (queue out=w356:refnum<queue>, error out=w355:errorcluster)  [unwired: 1 in, 1 out]
      }
    }
    n258 = local read "总磷总氮模块选择"() -> (w323:bool)
    n259 = case shown="假" w323 {
      tunnel: w326 -> [w345 w350]
      tunnel: w327 -> [w344 w349]
      tunnel: [w345 w348] -> w328
      tunnel: [w344 w347] -> w329
      frame False {
        w346 = FALSE ("通讯指示灯2")
        n260 = local write "总磷总氮通讯"(w346) -> ()
        n261 = local write "总磷总氮传感器状态显示"(w346) -> ()
      }
      frame True {
        n262 = Enqueue Element(queue=w350, element=cluster{"命令":string} {"命令"="总磷读取"} ("元素"), error in (no error)=w349) -> (queue out=w348:refnum<queue>, error out=w347:errorcluster)  [unwired: 1 in, 1 out]
      }
    }
    n263 = local read "CODMn选择"() -> (w324:bool)
    n264 = case shown="假" w324 {
      tunnel: w328 -> [w337 w342]
      tunnel: w329 -> [w336 w341]
      tunnel: [w337 w340] -> w330
      tunnel: [w336 w339] -> w331
      frame False {
        w338 = FALSE ("通讯指示灯3")
        n265 = local write "CODMn传感器状态显示"(w338) -> ()
        n266 = local write "CODMn通讯"(w338) -> ()
      }
      frame True {
        n267 = Enqueue Element(queue=w342, element=cluster{"命令":string} {"命令"="CODMn读取"} ("元素"), error in (no error)=w341) -> (queue out=w340:refnum<queue>, error out=w339:errorcluster)  [unwired: 1 in, 1 out]
      }
    }
    n268 = local read "CODCr选择"() -> (w325:bool)
    n269 = case shown="假" w325 {
      tunnel: w330 -> [_ w334]
      tunnel: w331 -> [_ w333]
      frame False {
        w332 = FALSE ("通讯指示灯3")
        n270 = local write "CODCr传感器状态显示"(w332) -> ()
        n271 = local write "CODCr通讯"(w332) -> ()
      }
      frame True {
        n272 = Enqueue Element(queue=w334, element=cluster{"命令":string} {"命令"="CODCr读取"} ("元素"), error in (no error)=w333) -> ()  [unwired: 1 in, 3 out]
      }
    }
  }
  n273 = while {
    tunnel: w88 -> [w368]
    tunnel: w76 -> [w367]
    tunnel: w67 -> [w362]
    tunnel: w64 -> [w366]
    tunnel: w61 -> [w365]
    tunnel: w51 -> [w364]
    tunnel: w42 -> [w363]
    tunnel: w31 -> [w361]
    tunnel: w30 -> [w360]
    stop <- FALSE stop-if-true
    # "氨氮站号是1，总磷总氮站号是2，CODMn站号是3，CODCr站号是4"
    n274 = event shown="[17] \"定时启动\": 值改变" {
      selector: _ -> [_ _ _ _ _ _ _ _ _ _ _ _ _ _ _ _ _ _ _ _ _ _ _ _ _]
      dyn-events: _ -> [_ _ _ _ _ _ _ _ _ _ _ _ _ _ _ _ _ _ _ _ _ _ _ _ _]
      timeout: _ -> [_ _ _ _ _ _ _ _ _ _ _ _ _ _ _ _ _ _ _ _ _ _ _ _ _]
      tunnel: w368 -> [_ _ _ _ _ _ _ _ _ _ w464 _ _ _ _ _ _ _ _ _ _ _ _ _ _]
      tunnel: w367 -> [_ _ _ _ _ _ _ _ _ _ _ w478 _ _ _ _ _ _ _ _ _ _ _ _ _]
      tunnel: w362 -> [_ _ _ _ _ _ _ _ _ _ _ _ _ w516 _ _ _ _ _ _ _ _ _ _ _]
      tunnel: w366 -> [_ _ _ _ _ _ _ _ _ _ _ _ _ _ _ _ _ _ _ w618 _ w709 w731 _ _]
      tunnel: w365 -> [_ _ _ _ _ _ _ _ _ _ _ _ _ _ _ _ _ _ _ _ _ _ w728 _ _]
      tunnel: w364 -> [_ _ _ _ _ _ _ _ _ _ _ _ w496 _ _ _ _ _ _ _ _ _ _ _ _]
      tunnel: [_ _ _ _ _ _ _ _ _ _ _ _ _ _ _ _ _ _ _ _ w643 _ _ _ _] -> _
      tunnel: w363 -> [_ _ _ _ _ _ _ _ _ _ _ _ _ _ w534 _ _ _ _ _ _ _ _ _ _]
      tunnel: w361 -> [_ _ _ _ _ _ _ _ _ _ _ _ _ _ _ _ w558 _ w608 _ _ _ _ _ _]
      tunnel: w360 -> [_ _ _ _ _ _ _ _ _ _ _ _ _ _ _ _ w557 _ w607 _ _ _ _ _ _]
      event Timeout {
        n275 = event-data() -> ()  [unwired: 1 in, 3 out]
      }
      event "氨氮量程", "氨氮检出限", "氨氮加标前水样浓度", "氨氮加标水杯定容体积", "氨氮母液浓度", "氨氮加标后水样浓度": Mouse Down {
        n276 = event-data() -> ("CtlRef"=w373:refnum<vi>)  [unwired: 1 in, 7 out]
        n277 = property class="DigNum (严格)"(reference=w373) -> (reference out=w371:refnum<vi>, "Value"=w372:dbl)  [unwired: 1 in, 1 out]
        n278 = call "数字键盘.vi"("OldNumber"=w372) -> ("NewNumber"=w370:sgl)
        n279 = property class="DigNum (严格)"(reference=w371, "Val(Sgnl)"=w370) -> ()  [unwired: 1 in, 2 out]
      }
      event "总磷母液浓度", "总磷加标水杯定容体积", "总磷加标后水样浓度", "总磷加标前水样浓度", "总磷检出限", "总磷量程": Mouse Down {
        n280 = event-data() -> ("CtlRef"=w377:refnum<vi>)  [unwired: 1 in, 7 out]
        n281 = property class="DigNum (严格)"(reference=w377) -> (reference out=w375:refnum<vi>, "Value"=w376:dbl)  [unwired: 1 in, 1 out]
        n282 = call "数字键盘.vi"("OldNumber"=w376) -> ("NewNumber"=w374:sgl)
        n283 = property class="DigNum (严格)"(reference=w375, "Val(Sgnl)"=w374) -> ()  [unwired: 1 in, 2 out]
      }
      event "总氮母液浓度", "总氮加标水杯定容体积", "总氮加标后水样浓度", "总氮加标前水样浓度", "总氮检出限", "总氮量程": Mouse Down {
        n284 = event-data() -> ("CtlRef"=w381:refnum<vi>)  [unwired: 1 in, 7 out]
        n285 = property class="DigNum (严格)"(reference=w381) -> (reference out=w379:refnum<vi>, "Value"=w380:dbl)  [unwired: 1 in, 1 out]
        n286 = call "数字键盘.vi"("OldNumber"=w380) -> ("NewNumber"=w378:sgl)
        n287 = property class="DigNum (严格)"(reference=w379, "Val(Sgnl)"=w378) -> ()  [unwired: 1 in, 2 out]
      }
      event "COD母液浓度", "COD加标水杯定容体积", "COD加标后水样浓度", "COD加标前水样浓度", "COD检出限", "COD量程": Mouse Down {
        n288 = event-data() -> ("CtlRef"=w385:refnum<vi>)  [unwired: 1 in, 7 out]
        n289 = property class="DigNum (严格)"(reference=w385) -> (reference out=w383:refnum<vi>, "Value"=w384:dbl)  [unwired: 1 in, 1 out]
        n290 = call "数字键盘.vi"("OldNumber"=w384) -> ("NewNumber"=w382:sgl)
        n291 = property class="DigNum (严格)"(reference=w383, "Val(Sgnl)"=w382) -> ()  [unwired: 1 in, 2 out]
      }
      event "CODCr检出限", "CODCr量程", "CODCr加标前水样浓度", "CODCr加标后水样浓度", "CODCr加标水杯定容体积", "CODCr母液浓度": Mouse Down {
        n292 = event-data() -> ("CtlRef"=w386:refnum<vi>)  [unwired: 1 in, 7 out]
        n293 = property class="DigNum (严格)"(reference=w386) -> (reference out=w388:refnum<vi>, "Value"=w389:dbl)  [unwired: 1 in, 1 out]
        n294 = call "数字键盘.vi"("OldNumber"=w389) -> ("NewNumber"=w387:sgl)
        n295 = property class="DigNum (严格)"(reference=w388, "Val(Sgnl)"=w387) -> ()  [unwired: 1 in, 2 out]
      }
      event "背隙补偿步数", "背隙补偿步数 2", "背隙补偿步数 3": Mouse Down {
        n296 = event-data() -> ("CtlRef"=w393:refnum<vi>)  [unwired: 1 in, 7 out]
        n297 = property class="DigNum (严格)"(reference=w393) -> (reference out=w392:refnum<vi>, "Value"=w391:i32)  [unwired: 1 in, 1 out]
        n298 = call "数字键盘.vi"("OldNumber"=w391) -> ("NewNumber"=w390:sgl)
        n299 = property class="DigNum (严格)"(reference=w392, "Val(Sgnl)"=w390) -> ()  [unwired: 1 in, 2 out]
      }
      event "背隙补偿步数", "背隙补偿步数 2", "背隙补偿步数 3": Value Change {
        w402 = "质控背隙补偿" ("section")
        n300 = event-data() -> ()  [unwired: 1 in, 6 out]
        n301 = call <vilib>:"Application Directory.vi"() -> ("Application Directory"=w409:path)
        n302 = Build Path(base path=w409, name or relative path="data\\Set.ini" ("名称或相对路径")) -> (appended path=w407:path)
        n303 = call <vilib>:"Open Config Data.vi"("configuration file path"=w407) -> ("error out"=w405:errorcluster, "refnum"=w406:T2)  [unwired: 8 in, 1 out]
        n304 = call-poly <vilib>:"Write Key.vi"("section"=w402, "error in (no error)"=w405, "value"="背隙补偿步数", "key"="背隙值1", "refnum"=w406) -> ("error out"=w396:errorcluster, "refnum out"=w399:T2)  [unwired: 4 in, 1 out]
        n305 = call-poly <vilib>:"Write Key.vi"("section"=w402, "error in (no error)"=w396, "value"="背隙补偿步数 2", "key"="背隙值2", "refnum"=w399) -> ("error out"=w397:errorcluster, "refnum out"=w398:T2)  [unwired: 4 in, 1 out]
        n306 = call-poly <vilib>:"Write Key.vi"("section"=w402, "error in (no error)"=w397, "value"="背隙补偿步数 3", "key"="背隙值3", "refnum"=w398) -> ()  [unwired: 4 in, 3 out]
      }
      event "氨氮模块", "总磷总氮模块选择", "CODMn选择", "CODCr选择": Value Change {
        w413 = "质控模块选择" ("section")
        n307 = event-data() -> ()  [unwired: 1 in, 6 out]
        n308 = call <vilib>:"Application Directory.vi"() -> ("Application Directory"=w431:path)
        n309 = Build Path(base path=w431, name or relative path="data\\Set.ini" ("名称或相对路径")) -> (appended path=w429:path)
        n310 = local read "氨氮模块"() -> (w419:bool)
        n311 = call <vilib>:"Open Config Data.vi"("configuration file path"=w429) -> ("error out"=w427:errorcluster, "refnum"=w428:T2)  [unwired: 8 in, 1 out]
        n312 = local read "总磷总氮模块选择"() -> (w418:bool)
        n313 = call-poly <vilib>:"Write Key.vi"("section"=w413, "error in (no error)"=w427, "value"=w419, "key"="模块1" ("section"), "refnum"=w428) -> ("error out"=w425:errorcluster, "refnum out"=w426:T2)  [unwired: 4 in, 1 out]
        n314 = local read "CODMn选择"() -> (w417:bool)
        n315 = call-poly <vilib>:"Write Key.vi"("section"=w413, "error in (no error)"=w425, "value"=w418, "key"="模块2" ("section"), "refnum"=w426) -> ("error out"=w423:errorcluster, "refnum out"=w424:T2)  [unwired: 4 in, 1 out]
        n316 = local read "CODCr选择"() -> (w410:bool)
        n317 = call-poly <vilib>:"Write Key.vi"("section"=w413, "error in (no error)"=w423, "value"=w417, "key"="模块3" ("section"), "refnum"=w424) -> ("error out"=w414:errorcluster, "refnum out"=w415:T2)  [unwired: 4 in, 1 out]
        n318 = call-poly <vilib>:"Write Key.vi"("section"=w413, "error in (no error)"=w414, "value"=w410, "key"="模块4" ("section"), "refnum"=w415) -> ("error out"=w411:errorcluster, "refnum out"=w412:T2)  [unwired: 4 in, 1 out]
        n319 = call <vilib>:"Close Config Data.vi"("error in (no error)"=w411, "refnum"=w412) -> ()  [unwired: 8 in, 2 out]
      }
      event "氨氮量程选择", "总氮量程选择", "总磷量程选择", "CODMn量程选择", "CODCr量程选择": Value Change {
        w438 = "质控模块量程选择" ("section")
        n320 = event-data() -> ()  [unwired: 1 in, 6 out]
        n321 = call <vilib>:"Application Directory.vi"() -> ("Application Directory"=w457:path)
        n322 = Build Path(base path=w457, name or relative path="data\\Set.ini" ("名称或相对路径")) -> (appended path=w455:path)
        n323 = local read "氨氮量程选择"() -> (w442:enum32{"H", "L", "AUTO"})
        n324 = call <vilib>:"Open Config Data.vi"("configuration file path"=w455) -> ("error out"=w453:errorcluster, "refnum"=w454:T2)  [unwired: 8 in, 1 out]
        n325 = local read "总氮量程选择"() -> (w441:enum32{"H", "L", "AUTO"})
        n326 = call-poly <vilib>:"Write Key.vi"("section"=w438, "error in (no error)"=w453, "value"=w442, "key"="氨氮" ("section"), "refnum"=w454) -> ("error out"=w451:errorcluster, "refnum out"=w452:T2)  [unwired: 4 in, 1 out]
        n327 = local read "总磷量程选择"() -> (w440:enum32{"H", "L", "AUTO"})
        n328 = call-poly <vilib>:"Write Key.vi"("section"=w438, "error in (no error)"=w451, "value"=w441, "key"="总氮" ("section"), "refnum"=w452) -> ("error out"=w449:errorcluster, "refnum out"=w450:T2)  [unwired: 4 in, 1 out]
        n329 = local read "CODMn量程选择"() -> (w439:enum32{"H", "L", "AUTO"})
        n330 = call-poly <vilib>:"Write Key.vi"("section"=w438, "error in (no error)"=w449, "value"=w440, "key"="总磷" ("section"), "refnum"=w450) -> ("error out"=w444:errorcluster, "refnum out"=w445:T2)  [unwired: 4 in, 1 out]
        n331 = local read "CODCr量程选择"() -> (w432:enum32{"H", "L", "AUTO"})
        n332 = call-poly <vilib>:"Write Key.vi"("section"=w438, "error in (no error)"=w444, "value"=w439, "key"="CODMn" ("section"), "refnum"=w445) -> ("error out"=w434:errorcluster, "refnum out"=w437:T2)  [unwired: 4 in, 1 out]
        n333 = call-poly <vilib>:"Write Key.vi"("section"=w438, "error in (no error)"=w434, "value"=w432, "key"="CODCr" ("section"), "refnum"=w437) -> ("error out"=w435:errorcluster, "refnum out"=w436:T2)  [unwired: 4 in, 1 out]
        n334 = call <vilib>:"Close Config Data.vi"("error in (no error)"=w435, "refnum"=w436) -> ()  [unwired: 8 in, 2 out]
      }
      event "氨氮量程", "氨氮检出限", "氨氮加标前水样浓度", "氨氮母液浓度", "氨氮加标水杯定容体积", "氨氮加标后水样浓度": Value Change {
        n335 = event-data() -> ()  [unwired: 1 in, 6 out]
        n336 = for {
          tunnel: w464 -> [w476] mode=indexing
          tunnel: [w475] -> w473 mode=indexing
          n337 = property class="DigNum (严格)"(reference=w476) -> ("Value"=w475:dbl)  [unwired: 1 in, 2 out]
        }
        n338 = Index Array(array=w473) -> (element #1=w472:dbl, element #2=w471:dbl, element #3=w458:dbl, element #4=w470:dbl, element #5=w469:dbl, element #6=w467:dbl)  [unwired: 6 in]
        n339 = global write "水样浓度全局.vi" "氨氮加标前水样浓度"(w458) -> ()
        n340 = Bundle By Name(cluster=T3 {"量程"=0.0, "检出限"=0.0, "加标前水样浓度"=0.0, "加标后水样浓度"=0.0, "加标水杯定容体积"=0.0, "加标母液浓度"=0.0, "加标体积"=0.0, "加标回收率"=0.0} ("参数"), "量程"=w472, "检出限"=w471, "加标前水样浓度"=w458, "加标后水样浓度"=w470, "加标水杯定容体积"=w469, "加标母液浓度"=w467) -> (w466:T3)
        n341 = call "加标回收率计算.vi"("参数"=w466) -> ("参数 out"=w465:T3)  [unwired: 10 in]
        n342 = call "质控参数保存.vi"("section"="氨氮质控参数", "参数"=w465) -> ()  [unwired: 9 in, 1 out]
        n343 = Unbundle By Name(w465) -> ("加标体积"=w459:dbl, "加标回收率"=w460:dbl)
        n344 = Index Array(array=w464, index #1=6 ("索引")) -> (element #1=w463:refnum<vi>, element #2=w461:refnum<vi>)  [unwired: 1 in]
        n345 = property class="DigNum (严格)"(reference=w463, "Value"=w459) -> ()  [unwired: 1 in, 2 out]
        n346 = property class="DigNum (严格)"(reference=w461, "Value"=w460) -> ()  [unwired: 1 in, 2 out]
      }
      event "总磷母液浓度", "总磷加标水杯定容体积", "总磷加标后水样浓度", "总磷加标前水样浓度", "总磷检出限", "总磷量程": Value Change {
        n347 = event-data() -> ()  [unwired: 1 in, 6 out]
        n348 = for {
          tunnel: w478 -> [w495] mode=indexing
          tunnel: [w494] -> w492 mode=indexing
          n349 = property class="DigNum (严格)"(reference=w495) -> ("Value"=w494:dbl)  [unwired: 1 in, 2 out]
        }
        n350 = Index Array(array=w492) -> (element #1=w491:dbl, element #2=w490:dbl, element #3=w477:dbl, element #4=w489:dbl, element #5=w488:dbl, element #6=w486:dbl)  [unwired: 6 in]
        n351 = global write "水样浓度全局.vi" "总磷加标前水样浓度"(w477) -> ()
        n352 = Bundle By Name(cluster=T3 {"量程"=0.0, "检出限"=0.0, "加标前水样浓度"=0.0, "加标后水样浓度"=0.0, "加标水杯定容体积"=0.0, "加标母液浓度"=0.0, "加标体积"=0.0, "加标回收率"=0.0} ("参数"), "量程"=w491, "检出限"=w490, "加标前水样浓度"=w477, "加标后水样浓度"=w489, "加标水杯定容体积"=w488, "加标母液浓度"=w486) -> (w485:T3)
        n353 = call "加标回收率计算.vi"("参数"=w485) -> ("参数 out"=w484:T3)  [unwired: 10 in]
        n354 = call "质控参数保存.vi"("section"="总磷质控参数", "参数"=w484) -> ()  [unwired: 9 in, 1 out]
        n355 = Unbundle By Name(w484) -> ("加标体积"=w481:dbl, "加标回收率"=w479:dbl)
        n356 = Index Array(array=w478, index #1=6 ("索引")) -> (element #1=w483:refnum<vi>, element #2=w480:refnum<vi>)  [unwired: 1 in]
        n357 = property class="DigNum (严格)"(reference=w483, "Value"=w481) -> ()  [unwired: 1 in, 2 out]
        n358 = property class="DigNum (严格)"(reference=w480, "Value"=w479) -> ()  [unwired: 1 in, 2 out]
      }
      event "总氮量程", "总氮检出限", "总氮加标前水样浓度", "总氮加标后水样浓度", "总氮加标水杯定容体积", "总氮母液浓度": Value Change {
        n359 = event-data() -> ()  [unwired: 1 in, 6 out]
        n360 = for {
          tunnel: w496 -> [w514] mode=indexing
          tunnel: [w513] -> w511 mode=indexing
          n361 = property class="DigNum (严格)"(reference=w514) -> ("Value"=w513:dbl)  [unwired: 1 in, 2 out]
        }
        n362 = Index Array(array=w511) -> (element #1=w510:dbl, element #2=w509:dbl, element #3=w497:dbl, element #4=w508:dbl, element #5=w507:dbl, element #6=w505:dbl)  [unwired: 6 in]
        n363 = global write "水样浓度全局.vi" "总氮加标前水样浓度"(w497) -> ()
        n364 = Bundle By Name(cluster=T3 {"量程"=0.0, "检出限"=0.0, "加标前水样浓度"=0.0, "加标后水样浓度"=0.0, "加标水杯定容体积"=0.0, "加标母液浓度"=0.0, "加标体积"=0.0, "加标回收率"=0.0} ("参数"), "量程"=w510, "检出限"=w509, "加标前水样浓度"=w497, "加标后水样浓度"=w508, "加标水杯定容体积"=w507, "加标母液浓度"=w505) -> (w504:T3)
        n365 = call "加标回收率计算.vi"("参数"=w504) -> ("参数 out"=w503:T3)  [unwired: 10 in]
        n366 = call "质控参数保存.vi"("section"="总氮质控参数", "参数"=w503) -> ()  [unwired: 9 in, 1 out]
        n367 = Unbundle By Name(w503) -> ("加标体积"=w500:dbl, "加标回收率"=w498:dbl)
        n368 = Index Array(array=w496, index #1=6 ("索引")) -> (element #1=w502:refnum<vi>, element #2=w499:refnum<vi>)  [unwired: 1 in]
        n369 = property class="DigNum (严格)"(reference=w502, "Value"=w500) -> ()  [unwired: 1 in, 2 out]
        n370 = property class="DigNum (严格)"(reference=w499, "Value"=w498) -> ()  [unwired: 1 in, 2 out]
      }
      event "COD母液浓度", "COD加标水杯定容体积", "COD加标后水样浓度", "COD加标前水样浓度", "COD检出限", "COD量程": Value Change {
        n371 = event-data() -> ()  [unwired: 1 in, 6 out]
        n372 = for {
          tunnel: w516 -> [w533] mode=indexing
          tunnel: [w532] -> w530 mode=indexing
          n373 = property class="DigNum (严格)"(reference=w533) -> ("Value"=w532:dbl)  [unwired: 1 in, 2 out]
        }
        n374 = Index Array(array=w530) -> (element #1=w529:dbl, element #2=w528:dbl, element #3=w515:dbl, element #4=w527:dbl, element #5=w526:dbl, element #6=w524:dbl)  [unwired: 6 in]
        n375 = global write "水样浓度全局.vi" "COD加标前水样浓度"(w515) -> ()
        n376 = Bundle By Name(cluster=T3 {"量程"=0.0, "检出限"=0.0, "加标前水样浓度"=0.0, "加标后水样浓度"=0.0, "加标水杯定容体积"=0.0, "加标母液浓度"=0.0, "加标体积"=0.0, "加标回收率"=0.0} ("参数"), "量程"=w529, "检出限"=w528, "加标前水样浓度"=w515, "加标后水样浓度"=w527, "加标水杯定容体积"=w526, "加标母液浓度"=w524) -> (w523:T3)
        n377 = call "加标回收率计算.vi"("参数"=w523) -> ("参数 out"=w522:T3)  [unwired: 10 in]
        n378 = call "质控参数保存.vi"("section"="COD质控参数", "参数"=w522) -> ()  [unwired: 9 in, 1 out]
        n379 = Unbundle By Name(w522) -> ("加标体积"=w519:dbl, "加标回收率"=w517:dbl)
        n380 = Index Array(array=w516, index #1=6 ("索引")) -> (element #1=w521:refnum<vi>, element #2=w518:refnum<vi>)  [unwired: 1 in]
        n381 = property class="DigNum (严格)"(reference=w521, "Value"=w519) -> ()  [unwired: 1 in, 2 out]
        n382 = property class="DigNum (严格)"(reference=w518, "Value"=w517) -> ()  [unwired: 1 in, 2 out]
      }
      event "CODCr母液浓度", "CODCr加标水杯定容体积", "CODCr加标前水样浓度", "CODCr检出限", "CODCr量程", "CODCr加标后水样浓度": Value Change {
        n383 = event-data() -> ()  [unwired: 1 in, 6 out]
        n384 = for {
          tunnel: w534 -> [w552] mode=indexing
          tunnel: [w551] -> w549 mode=indexing
          n385 = property class="DigNum (严格)"(reference=w552) -> ("Value"=w551:dbl)  [unwired: 1 in, 2 out]
        }
        n386 = Index Array(array=w549) -> (element #1=w548:dbl, element #2=w547:dbl, element #3=w535:dbl, element #4=w546:dbl, element #5=w545:dbl, element #6=w543:dbl)  [unwired: 6 in]
        n387 = global write "水样浓度全局.vi" "CODCr加标前水样浓度"(w535) -> ()
        n388 = Bundle By Name(cluster=T3 {"量程"=0.0, "检出限"=0.0, "加标前水样浓度"=0.0, "加标后水样浓度"=0.0, "加标水杯定容体积"=0.0, "加标母液浓度"=0.0, "加标体积"=0.0, "加标回收率"=0.0} ("参数"), "量程"=w548, "检出限"=w547, "加标前水样浓度"=w535, "加标后水样浓度"=w546, "加标水杯定容体积"=w545, "加标母液浓度"=w543) -> (w542:T3)
        n389 = call "加标回收率计算.vi"("参数"=w542) -> ("参数 out"=w541:T3)  [unwired: 10 in]
        n390 = call "质控参数保存.vi"("section"="CODCr质控参数", "参数"=w541) -> ()  [unwired: 9 in, 1 out]
        n391 = Unbundle By Name(w541) -> ("加标体积"=w538:dbl, "加标回收率"=w536:dbl)
        n392 = Index Array(array=w534, index #1=6 ("索引")) -> (element #1=w540:refnum<vi>, element #2=w537:refnum<vi>)  [unwired: 1 in]
        n393 = property class="DigNum (严格)"(reference=w540, "Value"=w538) -> ()  [unwired: 1 in, 2 out]
        n394 = property class="DigNum (严格)"(reference=w537, "Value"=w536) -> ()  [unwired: 1 in, 2 out]
      }
      event "手动调试": Value Change {
        n395 = event-data() -> ()  [unwired: 1 in, 6 out]
        n396 = call "手动调试界面.vi"() -> ()  [unwired: 16 in]
      }
      event "打开串口": Value Change {
        n397 = event-data() -> ()  [unwired: 1 in, 6 out]
        n398 = global read "断电保存全局.vi" "MB通信方式选择"() -> (w553:enum16{"串口", "TCP"})
        n399 = global read "断电保存全局.vi" "VISA Resource"() -> (w554:refnum<visa-resource-name>)
        n400 = global read "断电保存全局.vi" "PORT"() -> (w555:string)
        n401 = global read "断电保存全局.vi" "IP"() -> (w556:string)
        n402 = call "串口配置.vi"("PORT"=w555, "IP"=w556, "MB通信方式选择"=w553, "请选择串口:"=w554) -> ("PORT 2"=w560:string, "IP 2"=w561:string, "确认 2"=w563:bool, "VISA资源名称 2"=w562:refnum<visa-resource-name>, "MB通信方式选择 2"=w559:enum16{"串口", "TCP"})  [unwired: 3 in]
        n403 = case shown="真" w563 {
          tunnel: w562 -> [_ w569]
          tunnel: w558 -> [_ w568]
          tunnel: w561 -> [_ w567]
          tunnel: w560 -> [_ w566]
          tunnel: w559 -> [_ w565]
          tunnel: w557 -> [_ w564]
          frame False {
          }
          frame True {
            n404 = flat-sequence {
              tunnel: w569 -> [w573]
              tunnel: w568 -> [w575]
              tunnel: w567 -> [w572]
              tunnel: w566 -> [w571]
              tunnel: w565 -> [w570]
              tunnel: w564 -> [w574]
              frame #0 {
                n405 = global write "断电保存全局.vi" "IP"(w572) -> ()
                n406 = global write "断电保存全局.vi" "PORT"(w571) -> ()
                n407 = global write "断电保存全局.vi" "VISA Resource"(w573) -> ()
                n408 = global write "断电保存全局.vi" "MB通信方式选择"(w570) -> ()
                n409 = Enqueue Element(queue=w575, element=cluster{"命令":string} {"命令"="启用模块"} ("元素"), error in (no error)=w574) -> ()  [unwired: 1 in, 3 out]
              }
              frame #1 {
                n410 = call <vilib>:"Application Directory.vi"() -> ("Application Directory"=w590:path)
                n411 = Build Path(base path=w590, name or relative path="data\\sys.ini" ("名称或相对路径")) -> (appended path=w588:path)
                n412 = call <vilib>:"Open Config Data.vi"("configuration file path"=w588) -> ("error out"=w584:errorcluster, "refnum"=w587:T2)  [unwired: 8 in, 1 out]
                n413 = vi-ref "质控单元.lvlib:断电保存全局.vi"() -> (w586:refnum<vi>)
                n414 = call <userlib>:"Write Panel to INI__ogtk.vi"("error in (no error)"=w584, "VI ref"=w586, "refnum"=w587) -> ("error out"=w583:errorcluster, "refnum out"=w585:T2)  [unwired: 7 in]
                n415 = call <vilib>:"Close Config Data.vi"("error in (no error)"=w583, "refnum"=w585) -> ("error out"=w578:errorcluster, "file path"=w577:path)  [unwired: 8 in]
                n416 = Open/Create/Replace File(file path (use dialog)=w577, error in=w578) -> (refnum out=w581:refnum<file>, error out=w582:errorcluster)  [unwired: 4 in, 1 out]
                n417 = Flush File(refnum=w581, error in=w582) -> (refnum out=w580:refnum<file>, error out=w579:errorcluster)
                n418 = Close File(refnum=w580, error in=w579) -> ()  [unwired: 2 out]
              }
            }
          }
        }
      }
      event "定时启动": Value Change {
        n419 = event-data() -> ()  [unwired: 1 in, 6 out]
        n420 = flat-sequence {
          frame #0 {
            n421 = global read "断电保存全局.vi" "定时控制"() -> (w592:T8)
            n422 = call "周期设置.vi"("定时控制参数输入"=w592) -> ("定时控制参数输出"=w591:T9)  [unwired: 10 in]
            n423 = global write "断电保存全局.vi" "定时控制"(w591) -> ()
          }
          frame #1 {
            n424 = call <vilib>:"Application Directory.vi"() -> ("Application Directory"=w606:path)
            n425 = Build Path(base path=w606, name or relative path="data\\sys.ini" ("名称或相对路径")) -> (appended path=w604:path)
            n426 = call <vilib>:"Open Config Data.vi"("configuration file path"=w604) -> ("error out"=w600:errorcluster, "refnum"=w603:T2)  [unwired: 8 in, 1 out]
            n427 = vi-ref "质控单元.lvlib:断电保存全局.vi"() -> (w602:refnum<vi>)
            n428 = call <userlib>:"Write Panel to INI__ogtk.vi"("error in (no error)"=w600, "VI ref"=w602, "refnum"=w603) -> ("error out"=w599:errorcluster, "refnum out"=w601:T2)  [unwired: 7 in]
            n429 = call <vilib>:"Close Config Data.vi"("error in (no error)"=w599, "refnum"=w601) -> ("error out"=w594:errorcluster, "file path"=w593:path)  [unwired: 8 in]
            n430 = Open/Create/Replace File(file path (use dialog)=w593, error in=w594) -> (refnum out=w597:refnum<file>, error out=w598:errorcluster)  [unwired: 4 in, 1 out]
            n431 = Flush File(refnum=w597, error in=w598) -> (refnum out=w596:refnum<file>, error out=w595:errorcluster)
            n432 = Close File(refnum=w596, error in=w595) -> ()  [unwired: 2 out]
          }
        }
      }
      event "释放串口": Value Change {
        n433 = event-data() -> ()  [unwired: 1 in, 6 out]
        n434 = Two Button Dialog(message="确认是否释放串口，释放串口将导致通信失败！" ("消息")) -> (T button?=w609:bool)  [unwired: 2 in]
        n435 = case shown="真" w609 {
          tunnel: w608 -> [_ w612]
          tunnel: w607 -> [_ w611]
          frame False {
          }
          frame True {
            n436 = Bundle By Name(cluster=cluster{"命令":string} {"命令"=""} ("元素"), "命令"="停用模块" ("名称（未命名）")) -> (w613:cluster{"命令":string})
            n437 = Enqueue Element(queue=w612, element=w613, error in (no error)=w611) -> ()  [unwired: 1 in, 3 out]
          }
        }
      }
      event "加标回收": Value Change {
        n438 = event-data() -> ()  [unwired: 1 in, 6 out]
        n439 = Send Notification(notification=FALSE ("通知"), notifier=w618) -> ()  [unwired: 1 in, 2 out]
        n440 = call "质控启动流程对话框.vi"() -> ("确定启动"=w616:bool, "启动模块"=w621:T10, "直接启动"=w619:bool, "常规启动"=w620:bool)  [unwired: 8 in]
        n441 = case shown="真" w616 {
          tunnel: w621 -> [_ w630]
          tunnel: w620 -> [_ w629]
          tunnel: w619 -> [_ w628]
          frame False {
          }
          frame True {
            n442 = Bundle By Name(cluster=T5 {"是否启用仪器"=FALSE, "CODMn"={"启动测量模式"={"测量模式"=enum."水样测量"}, "确定按钮"=FALSE}, "启动模块"={"氨氮"=FALSE, "总磷"=FALSE, "总氮"=FALSE, "CODMn"=FALSE, "CODCr"=FALSE}, "常规启动"=FALSE, "直接启动"=FALSE} ("参数"), "是否启用仪器"=TRUE, "启动模块"=w630, "常规启动"=w629, "直接启动"=w628) -> (w622:T5)
            n443 = vi-ref "质控单元.lvlib:一体站流程质控自动启动.vi"() -> (w625:refnum<vi>)
            n444 = property class="VI"(reference=w625) -> ("Name"=w626:string, "Exec.State"=w624:T11)  [unwired: 1 in, 2 out]
            n445 = case shown="\"Idle\"" w624 {
              tunnel: w626 -> [_ w641]
              tunnel: w622 -> [_ w631]
              frame "Bad", Default {
              }
              frame "Idle" {
                n446 = Open VI Reference(type specifier VI Refnum (for type only)=refnum<vi> refnum ("类型说明符VI引用句柄（仅用于类型）"), vi path=w641, options=128 ("选项")) -> (vi reference=w642:refnum<vi>, error out=w638:errorcluster)  [unwired: 3 in]
                n447 = call-by-ref "开始异步调用"(reference=w642, error in=w638, "CODMn量程切换"="CODMn量程选择", "总磷量程切换"="总磷量程选择", "总氮量程切换"="总氮量程选择", "氨氮量程切换"="氨氮量程选择", "参数"=w631) -> (reference out=w640:refnum<vi>, error out=w639:errorcluster)  [unwired: 7 in]
                n448 = Close Reference(reference=w640, error in (no error)=w639) -> ()  [unwired: 1 out]
              }
            }
          }
        }
      }
      event "报警清除": Value Change {
        w649 = FALSE ("氨氮中断报警")
        n449 = event-data() -> ()  [unwired: 1 in, 6 out]
        n450 = global write "质控中断报警全局.vi" "氨氮中断报警"(w649) -> ()
        n451 = global write "质控中断报警全局.vi" "CODMn中断报警"(w649) -> ()
        n452 = global write "质控中断报警全局.vi" "总氮中断报警"(w649) -> ()
        n453 = global write "质控中断报警全局.vi" "总磷中断报警"(w649) -> ()
        n454 = global write "质控中断报警全局.vi" "CODCr中断报警"(w649) -> ()
        n455 = local read "氨氮模块"() -> (w659:bool)
        n456 = case shown="真" w659 {
          tunnel: [errorcluster {"status"=FALSE, "code"=0, "source"=""} ("error out") w702] -> w656
          frame False {
          }
          frame True {
            n457 = call "多个线圈写入.vi"("values"=bool[] [TRUE], "starting address"=u16 2106, "Slave ID"=u8 1) -> ("error out"=w702:errorcluster)  [unwired: 8 in]
          }
        }
        n458 = local read "总磷总氮模块选择"() -> (w658:bool)
        n459 = case shown="真" w658 {
          tunnel: w656 -> [w695 w698]
          tunnel: [w695 w696] -> w655
          frame False {
          }
          frame True {
            n460 = call "多个线圈写入.vi"("Error in"=w698, "values"=bool[] [TRUE], "starting address"=u16 2106, "Slave ID"=u8 2) -> ("error out"=w696:errorcluster)  [unwired: 7 in]
          }
        }
        n461 = local read "CODMn选择"() -> (w657:bool)
        n462 = case shown="真" w657 {
          tunnel: w655 -> [w689 w693]
          tunnel: [w689 w690] -> w646
          frame False {
          }
          frame True {
            n463 = call "多个线圈写入.vi"("Error in"=w693, "values"=bool[] [TRUE], "starting address"=u16 2106, "Slave ID"=u8 3) -> ("error out"=w690:errorcluster)  [unwired: 7 in]
          }
        }
        n464 = local read "CODCr选择"() -> (w647:bool)
        n465 = case shown="真" w647 {
          tunnel: w646 -> [w666 w670]
          tunnel: [w666 w667] -> w645
          frame False {
          }
          frame True {
            n466 = call "多个线圈写入.vi"("Error in"=w670, "values"=bool[] [TRUE], "starting address"=u16 2106, "Slave ID"=u8 4) -> ("error out"=w667:errorcluster)  [unwired: 7 in]
          }
        }
        n467 = local read "氨氮模块"() -> (w650:bool)
        n468 = case shown="真" w650 {
          tunnel: [w684 w685] -> w653
          tunnel: w645 -> [w684 _]
          frame False {
          }
          frame True {
            n469 = call "多个线圈写入.vi"("values"=bool[] [FALSE], "starting address"=u16 2106, "Slave ID"=u8 1) -> ("error out"=w685:errorcluster)  [unwired: 8 in]
          }
        }
        n470 = local read "总磷总氮模块选择"() -> (w651:bool)
        n471 = case shown="真" w651 {
          tunnel: w653 -> [w678 w681]
          tunnel: [w678 w679] -> w654
          frame False {
          }
          frame True {
            n472 = call "多个线圈写入.vi"("Error in"=w681, "values"=bool[] [FALSE], "starting address"=u16 2106, "Slave ID"=u8 2) -> ("error out"=w679:errorcluster)  [unwired: 7 in]
          }
        }
        n473 = local read "CODMn选择"() -> (w652:bool)
        n474 = case shown="真" w652 {
          tunnel: w654 -> [w672 w676]
          tunnel: [w672 w673] -> w644
          frame False {
          }
          frame True {
            n475 = call "多个线圈写入.vi"("Error in"=w676, "values"=bool[] [FALSE], "starting address"=u16 2106, "Slave ID"=u8 3) -> ("error out"=w673:errorcluster)  [unwired: 7 in]
          }
        }
        n476 = local read "CODCr选择"() -> (w648:bool)
        n477 = case shown="真" w648 {
          tunnel: w644 -> [w660 w664]
          tunnel: [w660 w661] -> w643
          frame False {
          }
          frame True {
            n478 = call "多个线圈写入.vi"("Error in"=w664, "values"=bool[] [FALSE], "starting address"=u16 2106, "Slave ID"=u8 4) -> ("error out"=w661:errorcluster)  [unwired: 7 in]
          }
        }
      }
      event "平行样测试": Value Change {
        n479 = event-data() -> ()  [unwired: 1 in, 6 out]
        n480 = Cancel Notification(0:w709) -> ()  [unwired: 1 in, 3 out]
        n481 = call "平行样启动流程对话框.vi"() -> ("启动模块"=w708:T12, "常规启动"=w706:bool, "确定启动"=w707:bool)  [unwired: 9 in]
        n482 = case shown="真" w707 {
          tunnel: w708 -> [_ w711]
          tunnel: w706 -> [_ w710]
          frame False {
          }
          frame True {
            (unwired) TRUE ("是否启用仪器")
            n483 = Bundle By Name(cluster=T6 {"参数启用"={"CODMn"=FALSE, "总磷"=FALSE, "总氮"=FALSE, "氨氮"=FALSE, "CODcr"=FALSE}, "采配水是否启动"=FALSE} ("参数"), "参数启用"=w711, "采配水是否启动"=w710) -> (w714:T6)
            n484 = vi-ref "一体站流程平行样自动启动.vi"() -> (w715:refnum<vi>)
            n485 = property class="VI"(reference=w715) -> ("Name"=w716:string, "Exec.State"=w713:T11)  [unwired: 1 in, 2 out]
            n486 = case shown="\"Idle\"" w713 {
              tunnel: w716 -> [_ w723]
              tunnel: w714 -> [_ w717]
              frame "Bad", Default {
              }
              frame "Idle" {
                n487 = Open VI Reference(type specifier VI Refnum (for type only)=refnum<vi> refnum ("类型说明符VI引用句柄（仅用于类型）"), vi path=w723, options=128 ("选项")) -> (vi reference=w724:refnum<vi>, error out=w722:errorcluster)  [unwired: 3 in]
                n488 = call-by-ref "开始异步调用"(reference=w724, error in=w722, "参数"=w717) -> (reference out=w719:refnum<vi>, error out=w718:errorcluster)  [unwired: 11 in]
                n489 = Close Reference(reference=w719, error in (no error)=w718) -> ()  [unwired: 1 out]
              }
            }
          }
        }
      }
      event "停止测量": Value Change {
        w725 = TRUE ("氨氮")
        # "停止采配水、氨氮、总磷总氮、COD、质控"
        n490 = event-data() -> ()  [unwired: 1 in, 6 out]
        n491 = Send Notification(notification=TRUE ("通知"), notifier=w731) -> ()  [unwired: 1 in, 2 out]
        n492 = call "质控启动参数选择对话框.vi"("CODCr"=w725, "CODMn"=w725, "总氮"=w725, "总磷"=w725, "氨氮"=w725) -> ("确定启动"=w726:bool, "启动模块"=w727:T10)  [unwired: 4 in, 1 out]
        n493 = case shown="真" w726 {
          tunnel: w727 -> [_ w738]
          frame False {
          }
          frame True {
            n494 = Unbundle By Name(w738) -> ("氨氮"=w736:bool, "总磷"=w735:bool, "总氮"=w734:bool, "CODMn"=w737:bool, "CODCr"=w732:bool)
            n495 = case shown="真" w737 {
              frame False {
              }
              frame True {
                n496 = call "CODMn停止命令 (子VI).vi"() -> ()  [unwired: 12 in]
                n497 = call "单个写入.vi"("value"=u16 2, "address"=u16 103, "Slave ID"=u8 3) -> ()  [unwired: 8 in, 1 out]
                n498 = Obtain Notifier(name (unnamed)="CODMn" ("名称（未命名）"), notification data type=FALSE) -> (notifier out=w771:refnum<notifier>)  [unwired: 2 in, 2 out]
                n499 = Send Notification(notification=TRUE ("通知"), notifier=w771) -> ()  [unwired: 1 in, 2 out]
              }
            }
            n500 = case shown="真" w732 {
              frame False {
              }
              frame True {
                n501 = call "CODCr停止命令 (子VI).vi"() -> ()  [unwired: 12 in]
                n502 = call "单个写入.vi"("value"=u16 2, "address"=u16 103, "Slave ID"=u8 4) -> ()  [unwired: 8 in, 1 out]
                n503 = Obtain Notifier(name (unnamed)="CODCr" ("名称（未命名）"), notification data type=FALSE) -> (notifier out=w742:refnum<notifier>)  [unwired: 2 in, 2 out]
                n504 = Send Notification(notification=TRUE ("通知"), notifier=w742) -> ()  [unwired: 1 in, 2 out]
              }
            }
            n505 = case shown="真" w736 {
              frame False {
              }
              frame True {
                n506 = call "单个写入.vi"("value"=u16 2, "address"=u16 103, "Slave ID"=u8 1) -> ()  [unwired: 8 in, 1 out]
                n507 = Obtain Queue(name (unnamed)="NH3N" ("名称（未命名）"), element data type=cluster{"命令":string, "data":variant} {"命令"="", "data"=variant}) -> (queue out=w767:refnum<queue>)  [unwired: 3 in, 2 out]
                n508 = Obtain Notifier(name (unnamed)="NH3N" ("名称（未命名）"), notification data type=FALSE) -> (notifier out=w763:refnum<notifier>)  [unwired: 2 in, 2 out]
                n509 = Send Notification(notification=TRUE ("通知"), notifier=w763) -> ()  [unwired: 1 in, 2 out]
                n510 = Enqueue Element(queue=w767, element=cluster{"命令":string, "data":variant} {"命令"="启动", "data"=variant(cluster{"站号":u16, "控制命令输出":u16[]} {"站号"=1, "控制命令输出"=[2816]})} ("元素")) -> ()  [unwired: 2 in, 3 out]
              }
            }
            n511 = Or(x=w735, y=w734) -> (x .or. y?=w733:bool)
            n512 = case shown="真" w733 {
              frame False {
              }
              frame True {
                n513 = call "单个写入.vi"("value"=u16 2, "address"=u16 103, "Slave ID"=u8 2) -> ()  [unwired: 8 in, 1 out]
                n514 = Obtain Queue(name (unnamed)="TP" ("名称（未命名）"), element data type=cluster{"命令":string, "data":variant} {"命令"="", "data"=variant}) -> (queue out=w756:refnum<queue>)  [unwired: 3 in, 2 out]
                n515 = Obtain Notifier(name (unnamed)="TNTP" ("名称（未命名）"), notification data type=FALSE) -> (notifier out=w752:refnum<notifier>)  [unwired: 2 in, 2 out]
                n516 = Send Notification(notification=TRUE ("通知"), notifier=w752) -> ()  [unwired: 1 in, 2 out]
                n517 = Enqueue Element(queue=w756, element=cluster{"命令":string, "data":variant} {"命令"="启动", "data"=variant(cluster{"站号":u16, "控制命令输出":u16[]} {"站号"=1, "控制命令输出"=[2816]})} ("元素")) -> ()  [unwired: 2 in, 3 out]
              }
            }
          }
        }
        n518 = Enqueue Element At Opposite End(queue=w728, element=T7 {"命令"="单个写入", {"starting address"=300, "holding register value"=2}} ("元素")) -> ()  [unwired: 2 in, 3 out]
      }
      event "查看": Value Change {
        n519 = event-data() -> ()  [unwired: 1 in, 6 out]
        n520 = property on="窗格" class="Pane"("Origin"=T1 {"Horizontal"=0, "Vertical"=640} ("原点")) -> ()  [unwired: 2 in, 2 out]
      }
      event "返回": Value Change {
        n521 = event-data() -> ()  [unwired: 1 in, 6 out]
        n522 = property on="窗格" class="Pane"("Origin"=T1 {"Horizontal"=0, "Vertical"=0} ("原点")) -> ()  [unwired: 2 in, 2 out]
      }
    }
  }
  n523 = call-by-ref "?"(reference=w37, error in=w39) -> (reference out=w41:refnum<vi>, error out=w40:errorcluster)  [unwired: 12 in]
  n524 = Open VI Reference(type specifier VI Refnum (for type only)=refnum<vi> refnum, vi path=w28, options=128 ("选项")) -> (vi reference=w26:refnum<vi>, error out=w24:errorcluster)  [unwired: 3 in]
  n525 = call-by-ref "?"(reference=w26, error in=w24) -> (reference out=w22:refnum<vi>, error out=w23:errorcluster)  [unwired: 12 in]
  n526 = Close Reference(reference=w41, error in (no error)=w40) -> ()  [unwired: 1 out]
  n527 = call-by-ref "?"(reference=w17, error in=w19, "CODMn"=w9, "总磷"=w10, "CODCr"=w13, "氨氮"=w11, "总氮"=w12) -> (reference out=w21:refnum<vi>, error out=w20:errorcluster)  [unwired: 7 in]
  n528 = Close Reference(reference=w22, error in (no error)=w23) -> ()  [unwired: 1 out]
  n529 = Close Reference(reference=w21, error in (no error)=w20) -> ()  [unwired: 1 out]
  n530 = vi-ref "质控单元.lvlib:周期启动 (子VI).vi"() -> (w8:refnum<vi>)
  n531 = property class="VI"(reference=w8) -> ("Name"=w7:string)  [unwired: 1 in, 2 out]
  n532 = Open VI Reference(type specifier VI Refnum (for type only)=refnum<vi> refnum, vi path=w7, options=128 ("选项")) -> (vi reference=w5:refnum<vi>, error out=w3:errorcluster)  [unwired: 3 in]
  n533 = call-by-ref "?"(reference=w5, error in=w3) -> (reference out=w1:refnum<vi>, error out=w2:errorcluster)  [unwired: 12 in]
  n534 = Close Reference(reference=w1, error in (no error)=w2) -> ()  [unwired: 1 out]
